vi "SpectrometerSpinCoater_v02_StreamMeasurement.vi"() -> ()   [LabVIEW 2020]
uses:
  <instrlib>/Classes/CCD/Abstract_CCD/Abstract_CCD.lvclass
  TypDef/DeviceQueue_Action.ctl
  TypDef/DeviceQueue_TypeDef.ctl
  TypDef/DataQueue_Action.ctl
  TypDef/DataQueue_TypeDef.ctl
  <instrlib>/Classes/CCD/Avantes/Avantes.lvclass
  <vilib>/Utility/error.llb/DialogType.ctl
  <vilib>/Instr/_visa.llb/VISA Configure Serial Port (Instr).vi
  TypDef/TabControl.ctl
panel:
  out "Arduino":bool
  out "NKT":bool
  out "Spectromter":bool
  in  "Abort Button":bool
  in  "Stop Button":bool
  in  "Tab Control":enum32{"Measure", "Settings"}(tab)
  out "Action":string
  in  "Preview":bool
  out "XY Graph":T1(graph)
  in  "Frames for Dark/Ref":dbl=1.0
  in  "StartSpin_Button":bool
  out "Overall Time":dbl
  in  "Seconds after Spin Stop":dbl[unit]=0.5
  in  "Program Spin Coater\nSpeed (rpm)          Time (s)":dbl[][](array[numeric])
  in  "Record RefSpec":bool
  in  "Record_Darkspec":bool
  in  "Comments":string="Just for testing"
  in  "File Name":string="Temp"
  in  "Save Path":path=path "C:/Users/Timo/Desktop/SpinCoater/Measurement"
  in  "Seconds to Spin Start":dbl[unit]=1.0
  in  "Calculate Frames":bool=TRUE
  in  "Frames":i32
  out "Frame Rate":dbl[unit]
  in  "Integration Time":dbl[unit]=3e-05
  in  "StartMeasurement_Button":bool
  in  "Speed":dbl
  in  "Milliseconds":dbl
  in  "Debug":bool
  in  "Port Arduino":refnum<visa-resource-name>="COM3"
  out "Error Arduino":bool caption="Error"
  in  "Init_Arduino":bool=TRUE caption="Init"
  out "Caption_Settings_Arduino":string="Arduino"
  out "Caption_Settings_NKT":string="NKT Laser"
  out "Error_Spectromter":bool caption="Error"
  in  "Init_Spectrometer":bool=TRUE caption="Init"
  out "Caption_Settings_Spectrometer":string="Spectromter"
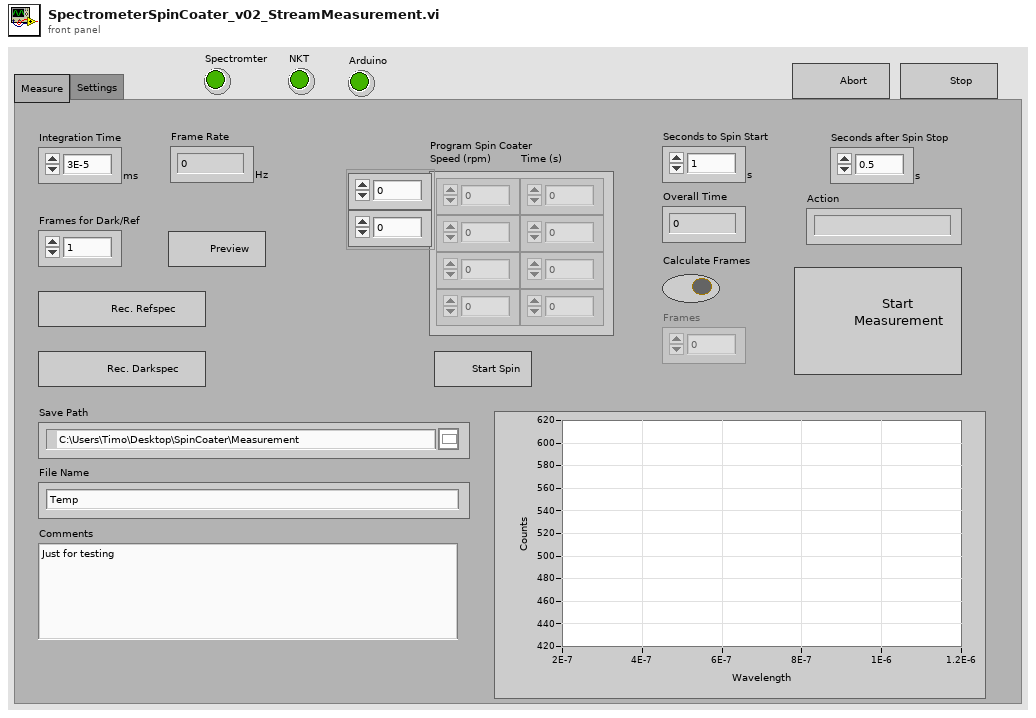
[diagram p1: front panel]
types:
  T1 = cluster{"Wavlength":dbl[unit][], "Image":dbl[]}[]
  T2 = cluster{"Dark":cluster{"Image":dbl[][][], "Frame Size":cluster{"F":i32, "Y":i32, "X":i32}}[], "Ref":cluster{"Image":dbl[][][], "Frame Size":cluster{"F":i32, "Y":i32, "X":i32}}[], "Wavlength":dbl[unit][], "spec":dbl[][]}
  T3 = cluster{"Port Arduino":refnum<visa-resource-name>, "Abstract_CCD.lvclass":refnum<class "Abstract_CCD.lvclass">}
  T4 = typedef "DataQueue_TypeDef.ctl" = cluster{"QueueAction":T5, "Data":cluster{"Image":dbl[][][], "Frame Size":cluster{"F":i32, "Y":i32, "X":i32}}[], "Data_Raw":cluster{"Image":dbl[][][], "Frame Size":cluster{"F":i32, "Y":i32, "X":i32}}[], "Data_Dark":cluster{"Image":dbl[][][], "Frame Size":cluster{"F":i32, "Y":i32, "X":i32}}[], "Data_Ref":cluster{"Image":dbl[][][], "Frame Size":cluster{"F":i32, "Y":i32, "X":i32}}[], "Device Information":string[], "Numeric Control":dbl, "Boolean":bool, "Wavelength":dbl[unit][], "Time":dbl[], "Time Stamp":timestamp, "Numeric Control 2":dbl, "TabControl":T6}
  T5 = typedef "DataQueue_Action.ctl" = enum16{"TimeOut", "Close_Program", "Abort", "Stop_Measurement", "Measure_InSituSpinCoating", "Measure_Spectrum", "Measure_SpectrumAdvanced", "Measure_SpectralStability", "Save_InSitu", "Save_SpectralStability", "Set_Ref", "Set_Dark", "Set_Wavelength", "Spectrometer_Measure", "Spectrometer_Preview", "Transfer_Settings"}
  T6 = typedef "TabControl.ctl" = enum16{"Measure", "Spectral Stability", "Settings"}
  T7 = typedef "DeviceQueue_TypeDef.ctl" = cluster{"QueueAction":T8, "Numeric 1":dbl, "Numeric 2":dbl, "Boolean 1":bool, "Boolean 2":bool, "Spin Program":dbl[][], "Spin Prg v07":cluster{"Speed (rpm)":dbl, "Time (s)":dbl, "Acc (rpm/s)":dbl}[], "Time Stamp":timestamp, "TabControl":T6}
  T8 = typedef "DeviceQueue_Action.ctl" = enum16{"TimeOut", "Wait", "Close_Program", "Abort", "Spectrometer_Init", "Spectrometer_Close", "Spectrometer_DeviceInformation", "Spectrometer_Measure", "Spectrometer_MeasureAdvanced", "Spectrometer_Preview", "Spectrometer_Abort", "Spectrometer_StartMeasurement", "Spectrometer_GetData", "Spectrometer_StopMeasurement", "Spectrometer_SetIntegrationTime", "Spectrometer_SetFrames", "Spectrometer_SetDarkspec", "Spectrometer_SetReference", "Spectrometer_SetTriggerMode", "Laser_Init", "Laser_Close", "Arduino_Init", "Arduino_Close", "Arduino_LoadProgram", "Arduino_StartProgram", "Arduino_SetSpeed", "Arduino_SetMillis", "Arduino_StopSpin", "Arduino_Shutter_SetPosition", "Arduino_Shutter_Close", "Arduino_Shutter_Open", "Measure_InSitu", "Measure_Spectrum", "Measure_InSituAdvanced", "Measure_SpectralStability", "Measure_Stop"}
  T9 = typedef "DataQueue_Action.ctl" = enum16{"TimeOut", "Close_Program", "Stop_Measurement", "Measure_InSituSpinCoating", "Save_Data", "Set_Ref", "Set_Dark", "Set_Wavelength", "Spectrometer_Measure", "Transfer_Settings"}
  T10 = enum16{"open", "replace", "create", "open or create", "replace or create", "replace or create with confirmation"}
  T11 = cluster{"Image":dbl[][][], "Frame Size":cluster{"F":i32, "Y":i32, "X":i32}}[]
  T12 = cluster{"Image":dbl[][][], "Frame Size":cluster{"F":i32, "Y":i32, "X":i32}}
  T13 = cluster{"Image":dbl[], "Image":dbl[], dbl[], "Numeric Control":dbl, "Numeric Control 2":dbl}
  T14 = typedef "DialogType.ctl" = u16
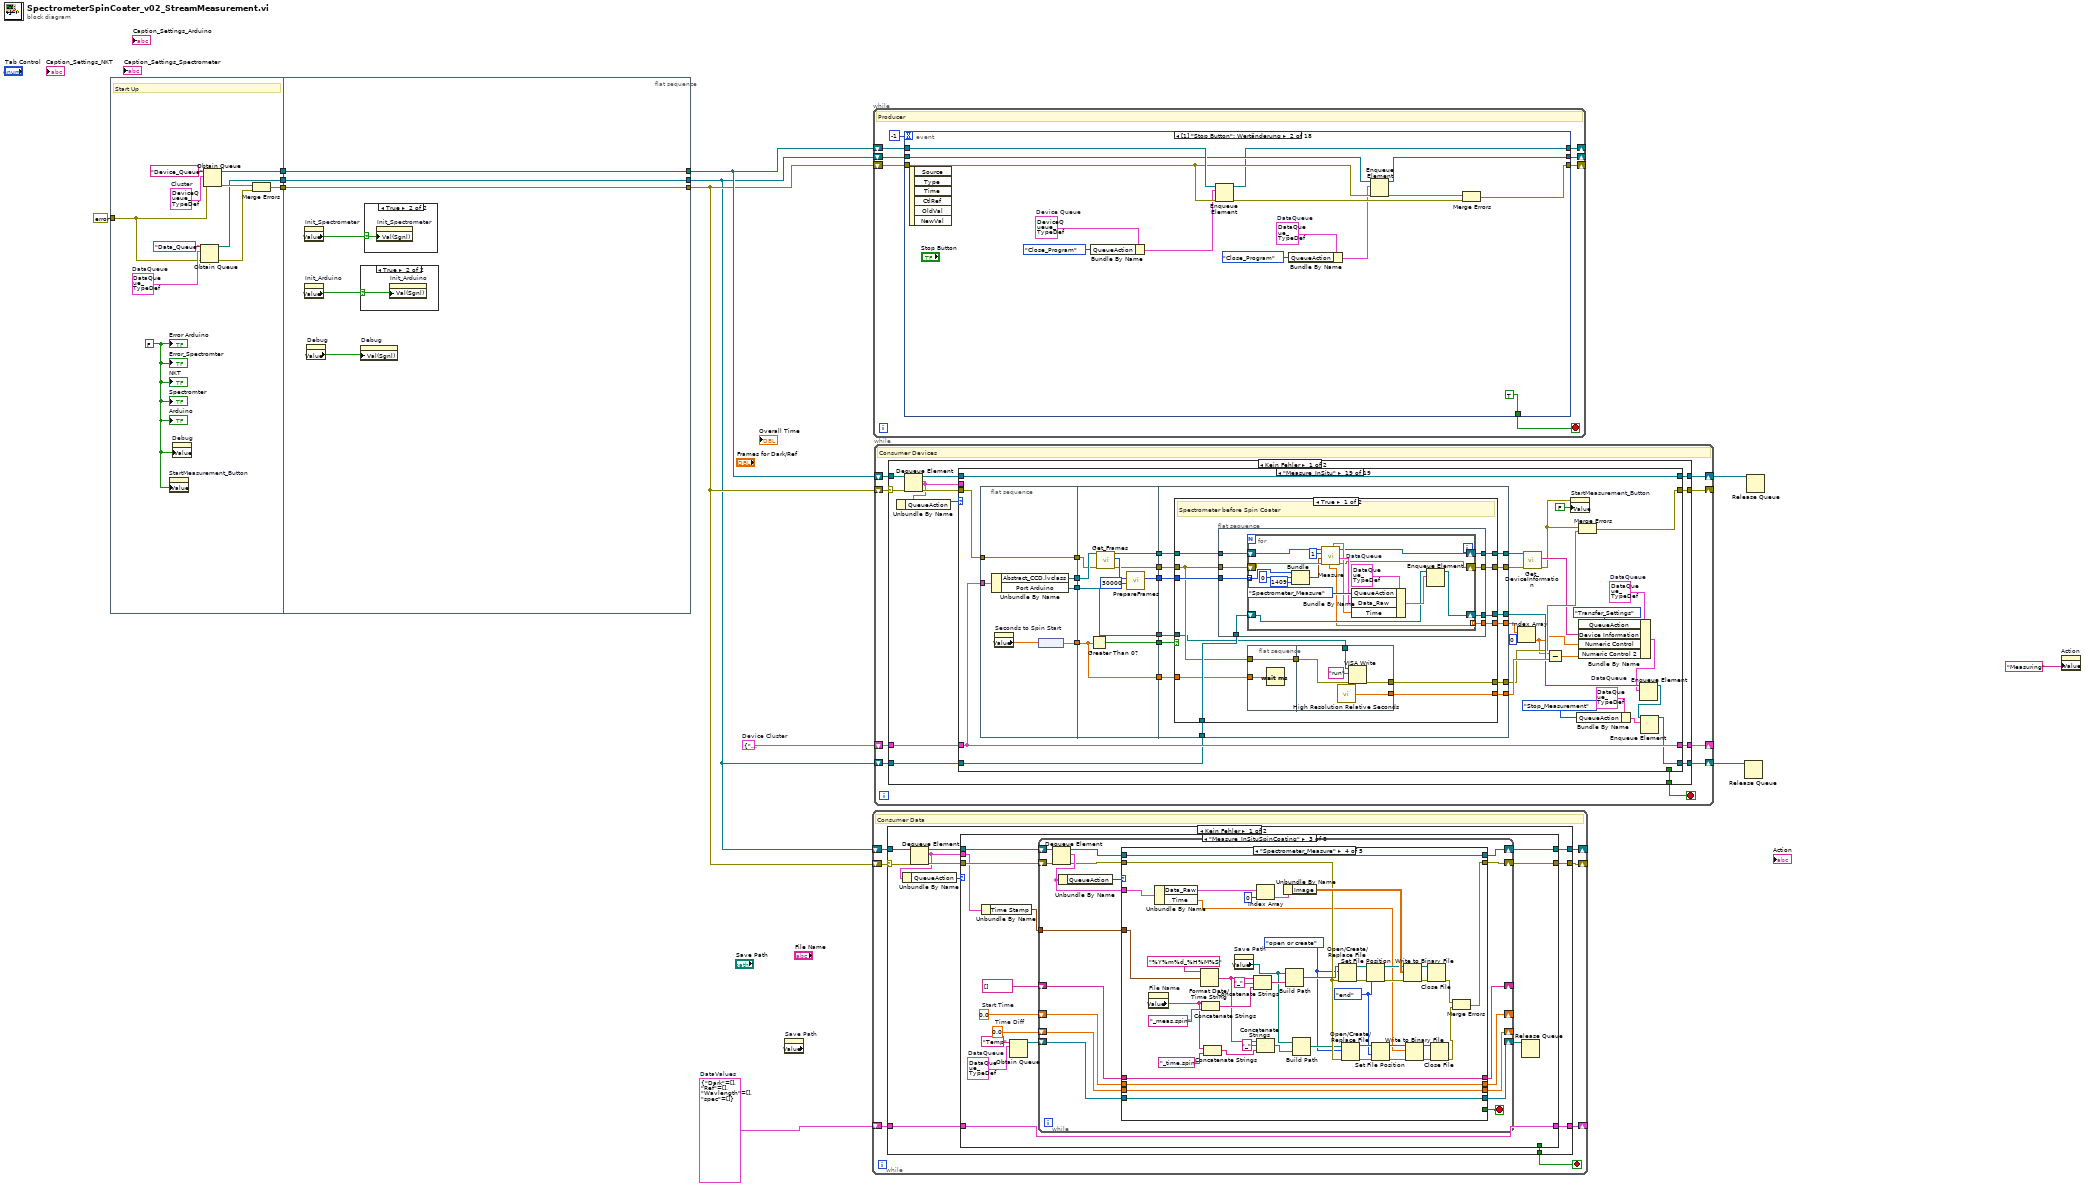
[diagram p0: block diagram]
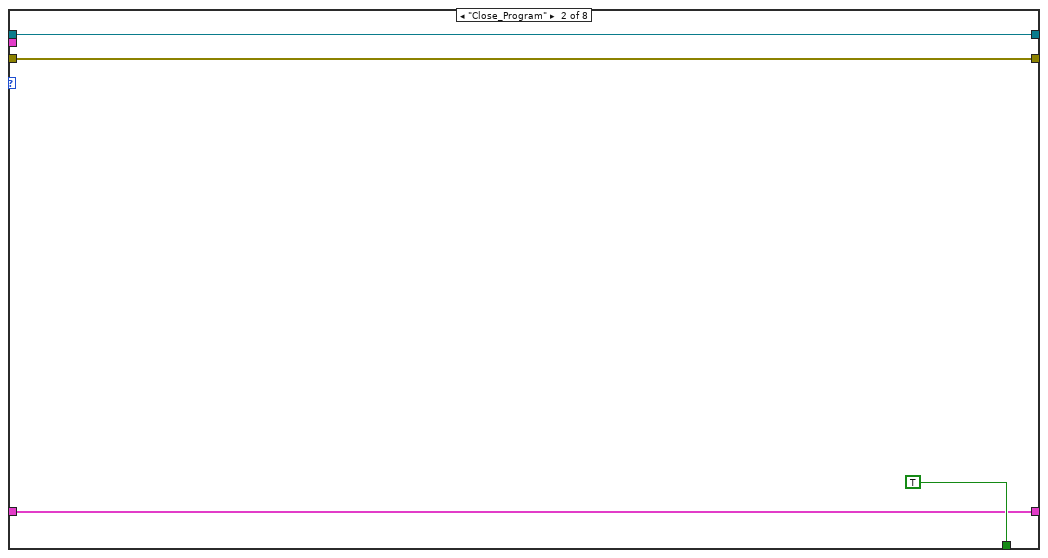
[diagram p5: hidden frame]
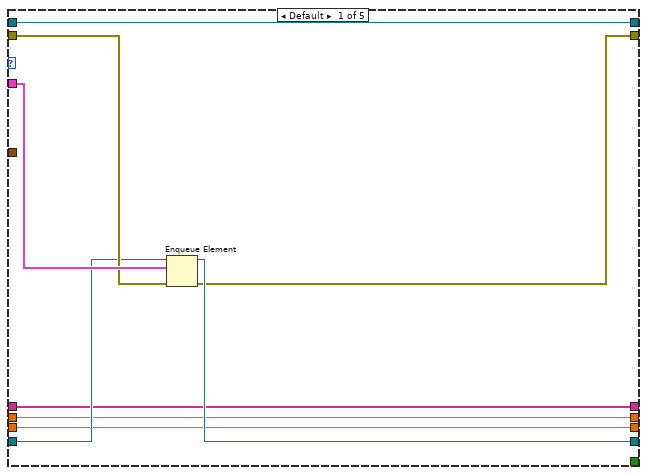
[diagram p6: hidden frame]
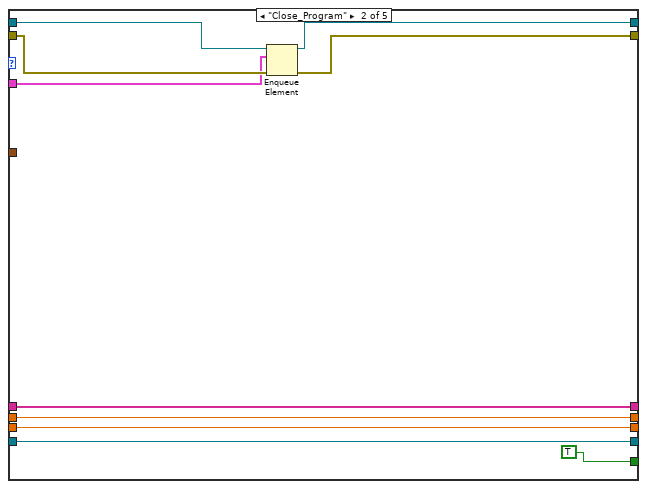
[diagram p7: hidden frame]
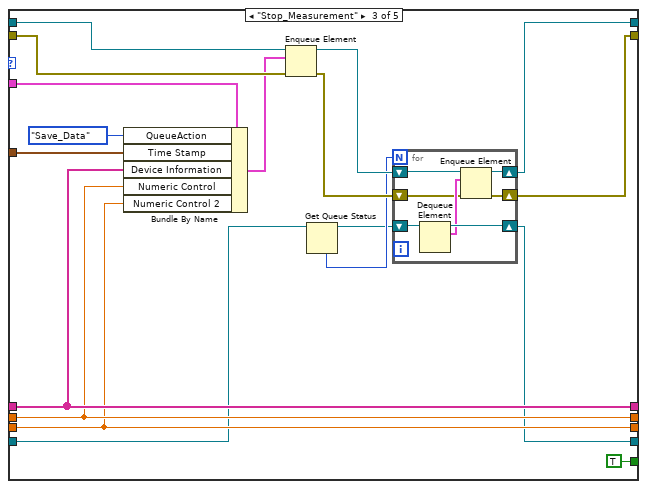
[diagram p8: hidden frame]
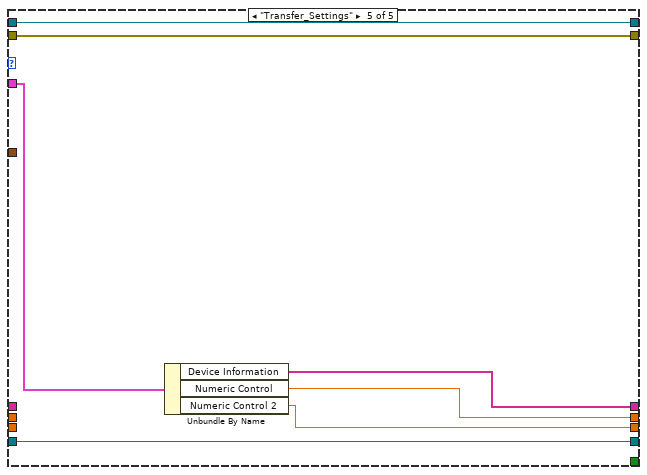
[diagram p9: hidden frame]
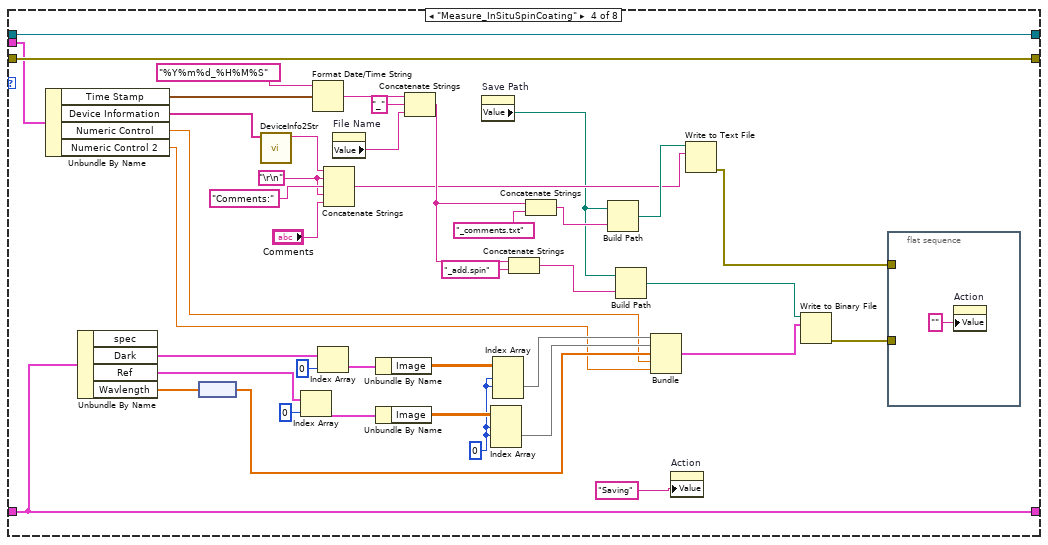
[diagram p10: hidden frame]
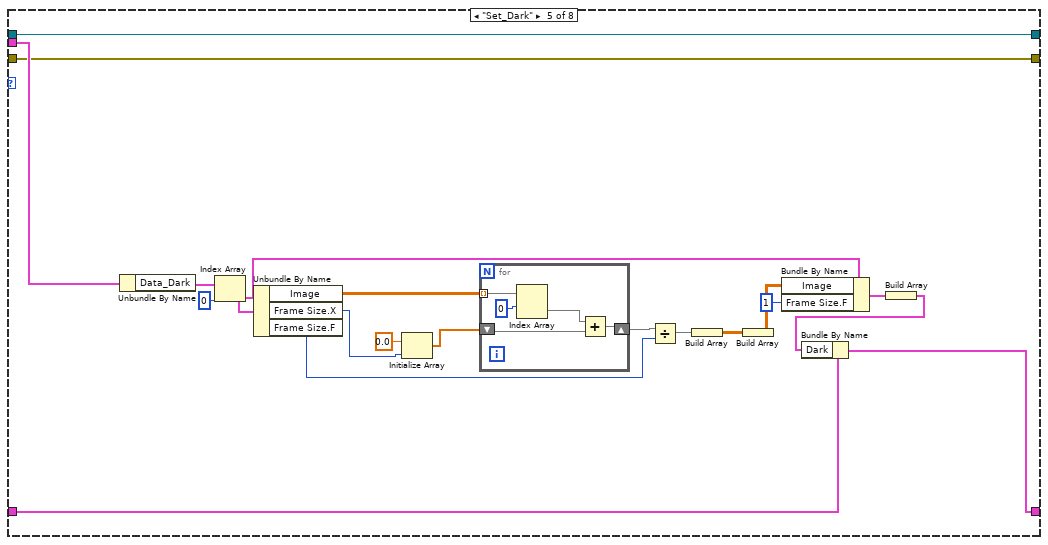
[diagram p11: hidden frame]
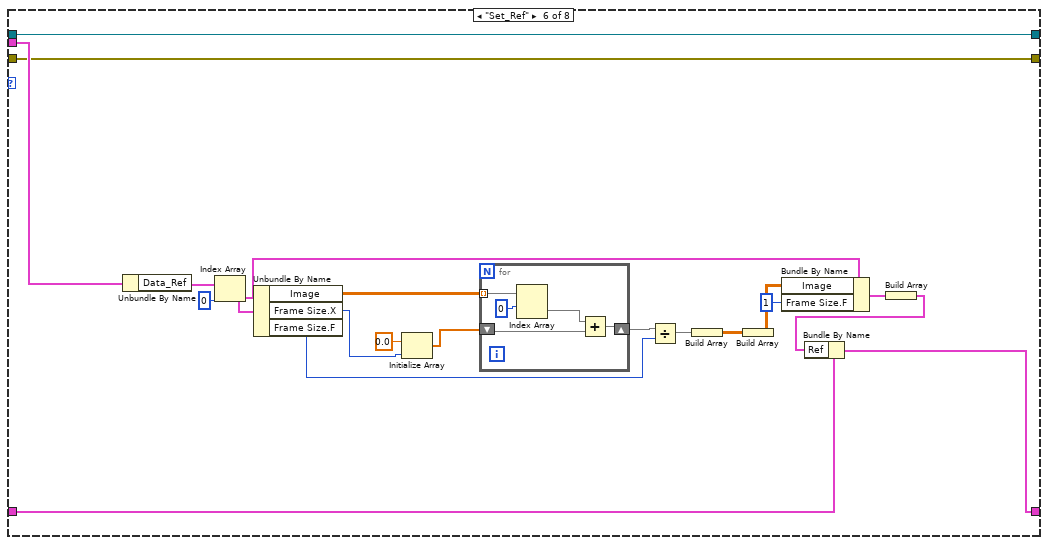
[diagram p12: hidden frame]
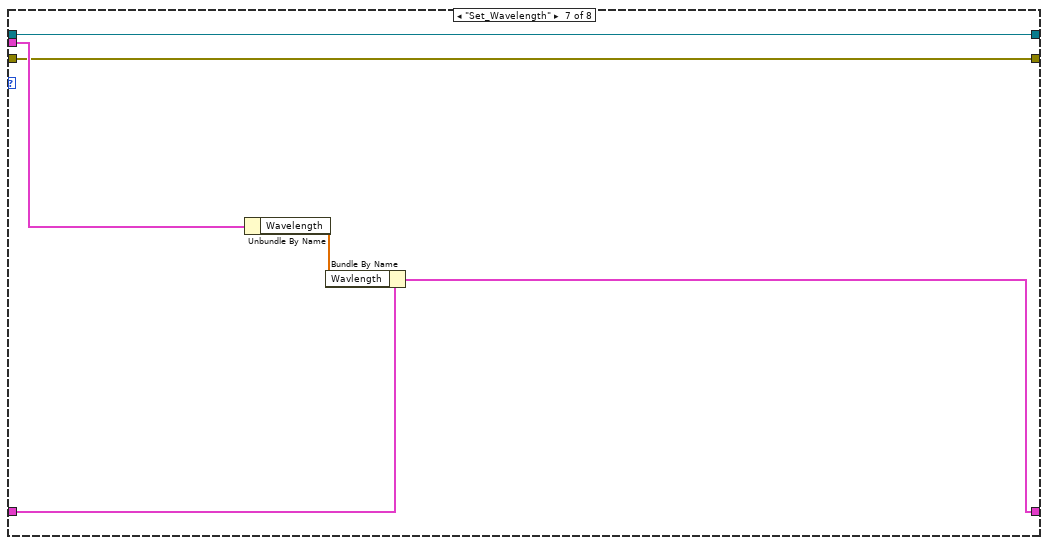
[diagram p13: hidden frame]
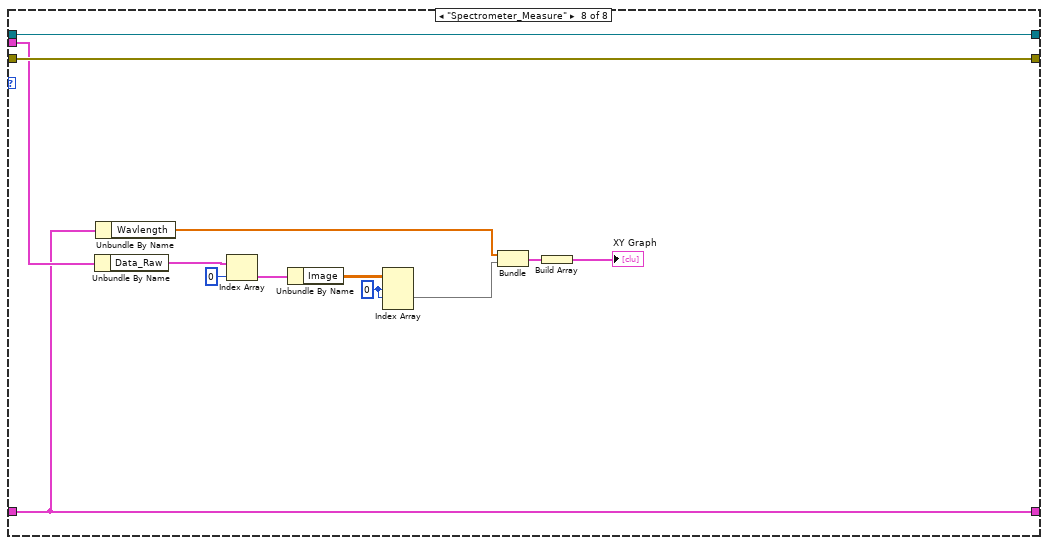
[diagram p14: hidden frame]
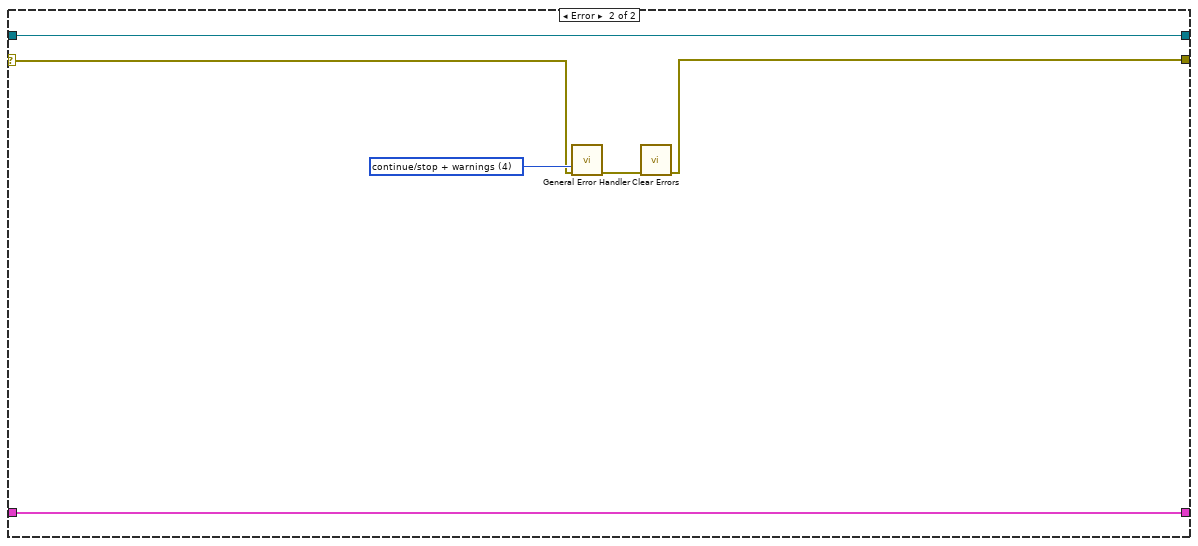
[diagram p15: hidden frame]
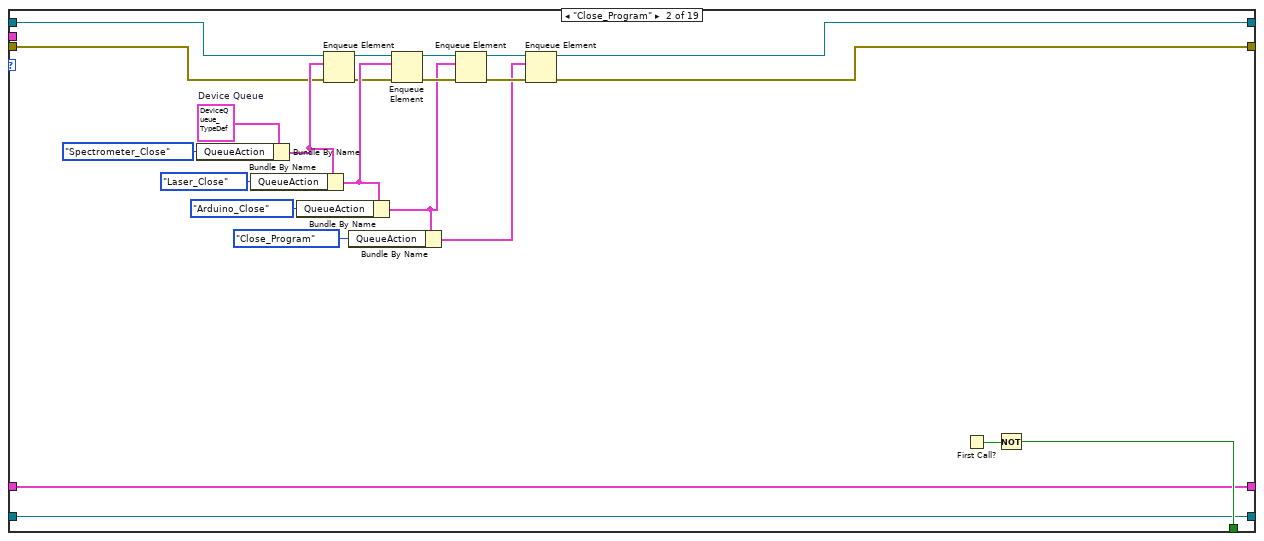
[diagram p17: hidden frame]
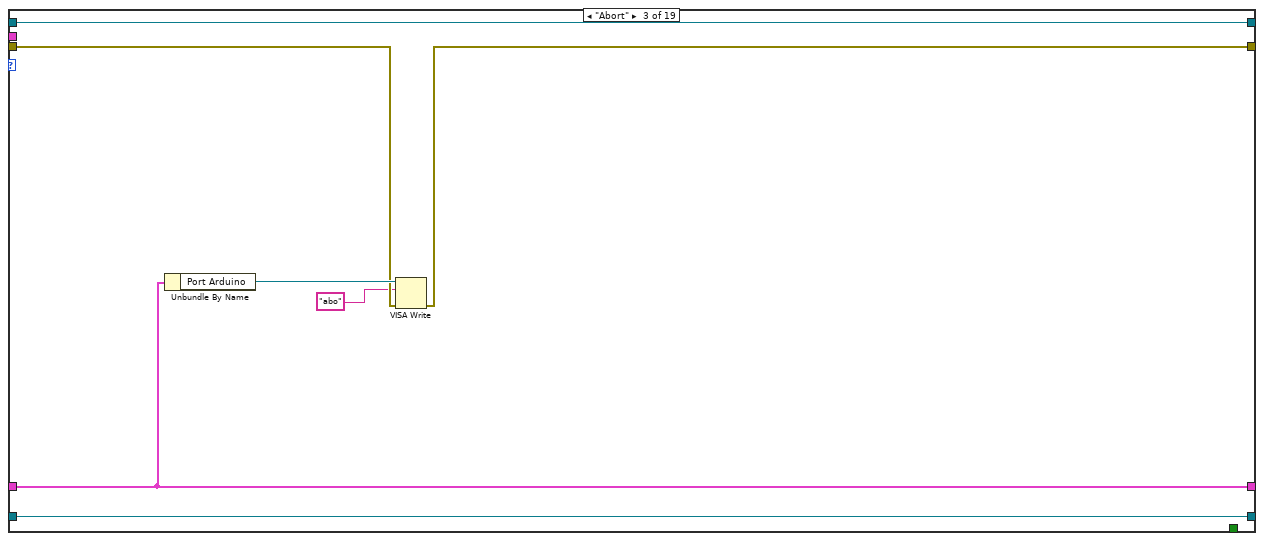
[diagram p18: hidden frame]
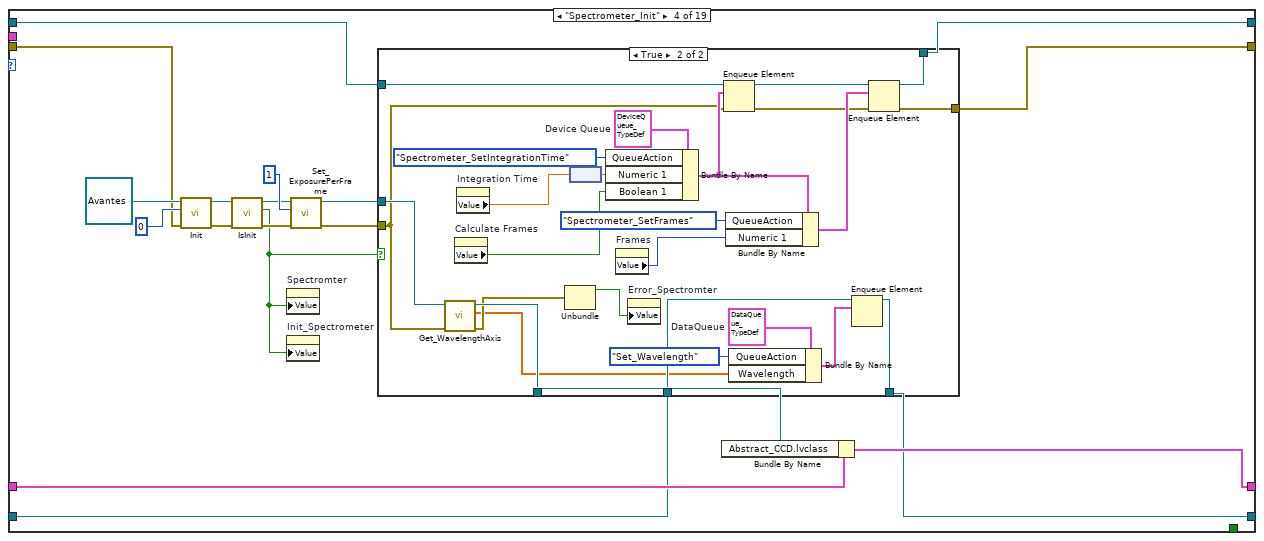
[diagram p19: hidden frame]
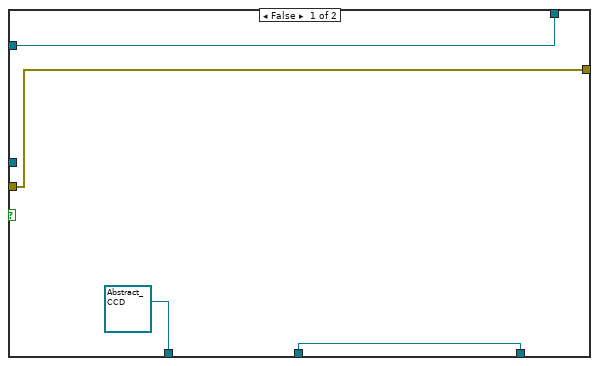
[diagram p20: hidden frame]
diagram:
  w2 = T2 {"Dark"=[], "Ref"=[], "Wavlength"=[], "spec"=[]}  # DataValues
  w7 = T3 {"Port Arduino"="", "Abstract_CCD.lvclass"=refnum}  # Device Cluster
  n1 = flat-sequence {
    tunnel: errorcluster {"status"=FALSE, "code"=0, "source"=""} ("error constant") -> [w18]
    tunnel: [w21] -> w11
    tunnel: [w15] -> w10
    tunnel: [w14] -> w9
    tunnel: w11 -> [w27]
    tunnel: w10 -> [w26]
    tunnel: w9 -> [w25]
    tunnel: [w27] -> w8
    tunnel: [w26] -> w3
    tunnel: [w25] -> w4
    frame #0 {
      w19 = T4 {"QueueAction"=enum."TimeOut", "Data"=[], "Data_Raw"=[], "Data_Dark"=[], "Data_Ref"=[], "Device Information"=[], "Numeric Control"=0.0, "Boolean"=FALSE, "Wavelength"=[], "Time"=[], "Time Stamp"=timestamp(0 s since 1904-01-01), "Numeric Control 2"=0.0, "TabControl"=enum."Measure"}  # DataQueue
      w22 = T7 {"QueueAction"=enum."TimeOut", "Numeric 1"=0.0, "Numeric 2"=0.0, "Boolean 1"=FALSE, "Boolean 2"=FALSE, "Spin Program"=[], "Spin Prg v07"=[], "Time Stamp"=timestamp(0 s since 1904-01-01), "TabControl"=enum."Measure"}  # Cluster
      w13 = FALSE ("Error Arduino")
      # "Start Up"
      n2 = property on="StartMeasurement_Button" class="Bool. (strikt)"("Value"=w13) -> ()  [unwired: 2 in, 2 out]
      n3 = property on="Debug" class="Bool. (strikt)"("Value"=w13) -> ()  [unwired: 2 in, 2 out]
      n4 = Obtain Queue(name (unnamed)="Data_Queue", element data type=w19, error in (no error)=w18) -> (queue out=w15:refnum<queue>, error out=w16:errorcluster)  [unwired: 2 in, 1 out]
      n5 = Obtain Queue(name (unnamed)="Device_Queue", element data type=w22, error in (no error)=w18) -> (queue out=w21:refnum<queue>, error out=w17:errorcluster)  [unwired: 2 in, 1 out]
      n6 = Merge Errors(w17, w16) -> (w14:errorcluster)
      "Error_Spectromter" <- w13
      "Error Arduino" <- w13
      "Spectromter" <- w13
      "NKT" <- w13
      "Arduino" <- w13
    }
    frame #1 {
      n7 = property on="Init_Spectrometer" class="Bool. (strikt)"() -> ("Value"=w29:bool)  [unwired: 2 in, 2 out]
      n8 = property on="Init_Arduino" class="Bool. (strikt)"() -> ("Value"=w28:bool)  [unwired: 2 in, 2 out]
      n9 = property on="Debug" class="Bool. (strikt)"() -> ("Value"=w24:bool)  [unwired: 2 in, 2 out]
      n10 = case shown="True" w28 {
        selector: w28 -> [_ w30]
        frame False {
        }
        frame True {
          n11 = property on="Init_Arduino" class="Bool. (strikt)"("Val(Sgnl)"=w30) -> ()  [unwired: 2 in, 2 out]
        }
      }
      n12 = property on="Debug" class="Bool. (strikt)"("Val(Sgnl)"=w24) -> ()  [unwired: 2 in, 2 out]
      n13 = case shown="True" w29 {
        selector: w29 -> [_ w31]
        frame False {
        }
        frame True {
          n14 = property on="Init_Spectrometer" class="Bool. (strikt)"("Val(Sgnl)"=w31) -> ()  [unwired: 2 in, 2 out]
        }
      }
    }
  }
  n15 = property on="Save Path" class="Pfad" props=["Value"]() -> ()  [unwired: 2 in, 3 out]
  n16 = while {
    shift-right: [w32] -> _
    shift-left: w4 -> [w38]
    shift-right: [w33] -> _
    shift-left: w3 -> [w37]
    shift-right: [w34] -> _
    shift-left: w2 -> [w36]
    stop <- w35 stop-if-true
    # "Consumer Data"
    n17 = case shown="Kein Fehler" w38 {
      selector: w38 -> [w49 w298]
      tunnel: w37 -> [w48 w299]
      tunnel: w36 -> [w46 w296]
      tunnel: [w45 _] -> w35
      tunnel: [w44 w296] -> w34
      tunnel: [w43 w299] -> w33
      tunnel: [w41 w297] -> w32
      frame No Error {
        n18 = Dequeue Element(queue=w48, error in (no error)=w49) -> (queue out=w42:refnum<queue>, element=w39:T4, error out=w40:errorcluster)  [unwired: 1 in, 1 out]
        n19 = Unbundle By Name(w39) -> ("QueueAction"=w47:T5)
        n20 = case shown="\"Measure_InSituSpinCoating\"" w47 {
          tunnel: w46 -> [w50 w55 w60 w194 w246 w271 w281 w292]
          tunnel: [_ TRUE _ _ _ _ _ _] -> w45
          tunnel: [w50 w55 w60 w194 w242 w267 w280 w292] -> w44
          tunnel: [w52 w54 w70 w225 w243 w268 w277 w295] -> w43
          tunnel: w42 -> [w52 w54 w68 w225 w243 w268 w277 w295]
          tunnel: [w51 w53 w69 w224 w244 w269 w278 w294] -> w41
          tunnel: w40 -> [w51 w53 w67 w224 w244 w269 w278 w294]
          tunnel: w39 -> [_ _ w62 w210 w245 w270 w279 w293]
          frame "TimeOut", Default {
          }
          frame "Close_Program" {
          }
          frame "Measure_InSituSpinCoating" {
            w58 = 0.0  # Time Diff
            w59 = 0.0  # Start Time
            w65 = T4 {"QueueAction"=enum."TimeOut", "Data"=[], "Data_Raw"=[], "Data_Dark"=[], "Data_Ref"=[], "Device Information"=[], "Numeric Control"=0.0, "Boolean"=FALSE, "Wavelength"=[], "Time"=[], "Time Stamp"=timestamp(0 s since 1904-01-01), "Numeric Control 2"=0.0, "TabControl"=enum."Measure"}  # DataQueue
            n21 = Unbundle By Name(w62) -> ("Time Stamp"=w61:timestamp)
            n22 = Obtain Queue(name (unnamed)="Temp", element data type=w65) -> (queue out=w64:refnum<queue>)  [unwired: 3 in, 2 out]
            n23 = while {
              shift-right: [w79] -> w70
              shift-left: w68 -> [w88]
              shift-right: [w80] -> w69
              shift-left: w67 -> [w87]
              shift-right: [w81] -> w63
              shift-left: w64 -> [w82]
              tunnel: w61 -> [w71]
              shift-right: [w74] -> _
              shift-left: w59 -> [w76]
              shift-right: [w75] -> _
              shift-left: w58 -> [w77]
              shift-right: [w72] -> _
              shift-left: string[] [] ("Device Information") -> [w73]
              stop <- w78 stop-if-true
              n24 = Dequeue Element(queue=w88, error in (no error)=w87) -> (queue out=w83:refnum<queue>, element=w85:T4, error out=w84:errorcluster)  [unwired: 1 in, 1 out]
              n25 = Unbundle By Name(w85) -> ("QueueAction"=w86:T5)
              n26 = case shown="\"Spectrometer_Measure\"" w86 {
                tunnel: w85 -> [w97 w105 w124 w170 w182]
                tunnel: w84 -> [w96 w106 w119 w149 w177]
                tunnel: w83 -> [w92 w107 w118 w167 w178]
                tunnel: w82 -> [w95 w102 w113 w138 w183]
                tunnel: [w94 w102 w110 w138 w183] -> w81
                tunnel: [w93 w103 w109 w139 w177] -> w80
                tunnel: [w92 w104 w108 w167 w178] -> w79
                tunnel: [_ TRUE TRUE _ _] -> w78
                tunnel: w77 -> [w89 w99 w120 w134 _]
                tunnel: w76 -> [w90 w100 w121 w135 _]
                tunnel: [w89 w99 w120 w134 w179] -> w75
                tunnel: [w90 w100 w121 w135 w180] -> w74
                tunnel: w73 -> [w91 w98 w122 w136 _]
                tunnel: [w91 w98 w122 w136 w181] -> w72
                tunnel: w71 -> [_ _ w123 w172 _]
                frame Default {
                  n27 = Enqueue Element(queue=w95, element=w97, error in (no error)=w96) -> (queue out=w94:refnum<queue>, error out=w93:errorcluster)  [unwired: 1 in, 1 out]
                }
                frame "Close_Program" {
                  n28 = Enqueue Element(queue=w107, element=w105, error in (no error)=w106) -> (queue out=w104:refnum<queue>, error out=w103:errorcluster)  [unwired: 1 in, 1 out]
                }
                frame "Stop_Measurement" {
                  n29 = Bundle By Name(cluster=w124, "QueueAction"=DataQueue_Action."Save_Data", "Time Stamp"=w123, "Device Information"=w122, "Numeric Control"=w121, "Numeric Control 2"=w120) -> (w117:T4)
                  n30 = Enqueue Element(queue=w118, element=w117, error in (no error)=w119) -> (queue out=w115:refnum<queue>, error out=w114:errorcluster)  [unwired: 1 in, 1 out]
                  n31 = Get Queue Status(queue=w113) -> (queue out=w111:refnum<queue>, # elements in queue=w112:i32)  [unwired: 2 in, 6 out]
                  n32 = for {
                    N: w112 -> [_]
                    shift-right: [w131] -> w110
                    shift-left: w111 -> [w132]
                    shift-right: [w128] -> w108
                    shift-left: w115 -> [w129]
                    shift-right: [w126] -> w109
                    shift-left: w114 -> [w127]
                    n33 = Dequeue Element(queue=w132) -> (queue out=w131:refnum<queue>, element=w130:T4)  [unwired: 2 in, 2 out]
                    n34 = Enqueue Element(queue=w129, element=w130, error in (no error)=w127) -> (queue out=w128:refnum<queue>, error out=w126:errorcluster)  [unwired: 1 in, 1 out]
                  }
                }
                frame "Spectrometer_Measure" {
                  w133 = T10."open or create" ("operation (0:open)")
                  w137 = enum16{"start", "end", "current"}."end" ("from (0:start)")
                  n35 = property on="File Name" class="Str"() -> ("Value"=w169:string)  [unwired: 2 in, 2 out]
                  n36 = Unbundle By Name(w170) -> ("Data_Raw"=w160:T11, "Time"=w148:dbl[])
                  n37 = Format Date/Time String(time format string (%c)="%Y%m%d_%H%M%S", seconds (now)=w172) -> (date/time string=w147:string)  [unwired: 1 in]
                  n38 = Concatenate Strings(w169, "_meas.spin" ("string")) -> (w173:string)
                  n39 = Concatenate Strings(w169, "_time.spin" ("string")) -> (w145:string)
                  n40 = property on="Save Path" class="Pfad"() -> ("Value"=w143:path)  [unwired: 2 in, 2 out]
                  n41 = Concatenate Strings(w147, "_" ("string"), w173) -> (w171:string)
                  n42 = Index Array(array=w160, index=0) -> (element=w159:T12)
                  n43 = Concatenate Strings(w147, "_" ("string"), w145) -> (w144:string)
                  n44 = Unbundle By Name(w159) -> ("Image"=w157:dbl[][][])
                  n45 = Build Path(base path=w143, name or relative path=w171) -> (appended path=w150:path)
                  n46 = Build Path(base path=w143, name or relative path=w144) -> (appended path=w142:path)
                  n47 = Open/Create/Replace File(file path (use dialog)=w150, error in=w149, operation (0:open)=w133) -> (refnum out=w152:refnum<file>, error out=w151:errorcluster)  [unwired: 3 in, 1 out]
                  n48 = Open/Create/Replace File(file path (use dialog)=w142, error in=w149, operation (0:open)=w133) -> (refnum out=w166:refnum<file>, error out=w161:errorcluster)  [unwired: 3 in, 1 out]
                  n49 = Set File Position(refnum=w152, from (0:start)=w137, error in=w151) -> (refnum out=w156:refnum<file>, error out=w155:errorcluster)  [unwired: 1 in]
                  n50 = Set File Position(refnum=w166, from (0:start)=w137, error in=w161) -> (refnum out=w165:refnum<file>, error out=w162:errorcluster)  [unwired: 1 in]
                  n51 = Write to Binary File(file (use dialog)=w156, data=w157, error in=w155) -> (refnum out=w153:refnum<file>, error out=w154:errorcluster)  [unwired: 3 in, 1 out]
                  n52 = Write to Binary File(file (use dialog)=w165, data=w148, error in=w162) -> (refnum out=w164:refnum<file>, error out=w163:errorcluster)  [unwired: 3 in, 1 out]
                  n53 = Close File(refnum=w153, error in=w154) -> (error out=w141:errorcluster)  [unwired: 1 out]
                  n54 = Close File(refnum=w164, error in=w163) -> (error out=w140:errorcluster)  [unwired: 1 out]
                  n55 = Merge Errors(w141, w140) -> (w139:errorcluster)
                }
                frame "Transfer_Settings" {
                  n56 = Unbundle By Name(w182) -> ("Device Information"=w181:string[], "Numeric Control"=w180:dbl, "Numeric Control 2"=w179:dbl)
                }
              }
            }
            n57 = Release Queue(queue=w63) -> ()  [unwired: 2 in, 3 out]
          }
          frame "Measure_InSituSpinCoating" {
            w196 = "\r\n"
            w214 = 0 ("index (page)")
            n58 = Unbundle By Name(w210) -> ("Time Stamp"=w208:timestamp, "Device Information"=w199:string[], "Numeric Control"=w193:dbl, "Numeric Control 2"=w192:dbl)
            n59 = Unbundle By Name(w194) -> ("Dark"=w221:T11, "Ref"=w219:T11, "Wavlength"=w223:dbl[unit][])  [unwired: 1 out]
            n60 = node(w223) -> (w211:dbl[])
            n61 = call "DeviceInfo2Str.vi"("Device Information"=w199) -> ("String"=w198:string)  [unwired: 10 in]
            n62 = Index Array(array=w219, index=0) -> (element=w217:T12)
            n63 = Format Date/Time String(time format string (%c)="%Y%m%d_%H%M%S", seconds (now)=w208) -> (date/time string=w207:string)  [unwired: 1 in]
            n64 = Index Array(array=w221, index=0) -> (element=w218:T12)
            n65 = Concatenate Strings(w198, w196, "Comments:" ("string"), w196, "Comments") -> (w191:string)
            n66 = property on="File Name" class="Str"() -> ("Value"=w189:string)  [unwired: 2 in, 2 out]
            n67 = Unbundle By Name(w218) -> ("Image"=w216:dbl[][][])
            n68 = Unbundle By Name(w217) -> ("Image"=w215:dbl[][][])
            n69 = Concatenate Strings(w207, "_" ("string"), w189) -> (w205:string)
            n70 = property on="Save Path" class="Pfad"() -> ("Value"=w188:path)  [unwired: 2 in, 2 out]
            n71 = Index Array(array=w215, index (dim 0)=w214, index (dim 1)=w214) -> (element=w212:dbl[])  [unwired: 1 in]
            n72 = Index Array(array=w216, index (dim 0)=w214, index (dim 1)=w214) -> (element=w213:dbl[])  [unwired: 1 in]
            n73 = Concatenate Strings(w205, "_add.spin" ("string")) -> (w203:string)
            n74 = Concatenate Strings(w205, "_comments.txt" ("string")) -> (w202:string)
            n75 = Build Path(base path=w188, name or relative path=w202) -> (appended path=w201:path)
            n76 = Build Path(base path=w188, name or relative path=w203) -> (appended path=w187:path)
            n77 = Bundle("Image"=w213, "Image"=w212, w211, "Numeric Control"=w193, "Numeric Control 2"=w192) -> (w186:T13)  [unwired: 1 in]
            n78 = property on="Action" class="Str"("Value"="Saving" ("Action")) -> ()  [unwired: 2 in, 2 out]
            n79 = Write to Text File(file (use dialog)=w201, text=w191) -> (error out=w185:errorcluster)  [unwired: 2 in, 2 out]
            n80 = Write to Binary File(file (use dialog)=w187, data=w186) -> (error out=w184:errorcluster)  [unwired: 4 in, 2 out]
            n81 = flat-sequence {
              tunnel: w185 -> [_]
              tunnel: w184 -> [_]
              frame #0 {
                n82 = property on="Action" class="Str"("Value"="" ("Action")) -> ()  [unwired: 2 in, 2 out]
              }
            }
          }
          frame "Set_Dark" {
            n83 = Unbundle By Name(w245) -> ("Data_Dark"=w232:T11)
            n84 = Index Array(array=w232, index=0) -> (element=w231:T12)
            n85 = Unbundle By Name(w231) -> ("Image"=w240:dbl[][][], "Frame Size.X"=w238:i32, "Frame Size.F"=w235:i32)
            n86 = Initialize Array(0.0 ("element"), w238) -> (w237:dbl[])
            n87 = for {
              tunnel: w240 -> [w251] mode=indexing
              shift-right: [w247] -> w236
              shift-left: w237 -> [w248]
              n88 = Index Array(array=w251, index (row)=0) -> (element=w249:dbl[])  [unwired: 1 in]
              n89 = Add(x=w249, y=w248) -> (x+y=w247:dbl[])
            }
            n90 = Divide(x=w236, y=w235) -> (x/y=w234:dbl[])
            n91 = Build Array(w234) -> (w233:dbl[][])
            n92 = Build Array(w233) -> (w230:dbl[][][])
            n93 = Bundle By Name(cluster=w231, "Image"=w230, "Frame Size.F"=1) -> (w228:T12)
            n94 = Build Array(w228) -> (w227:T11)
            n95 = Bundle By Name(cluster=w246, "Dark"=w227) -> (w242:T2)
          }
          frame "Set_Ref" {
            n96 = Unbundle By Name(w270) -> ("Data_Ref"=w257:T11)
            n97 = Index Array(array=w257, index=0) -> (element=w256:T12)
            n98 = Unbundle By Name(w256) -> ("Image"=w265:dbl[][][], "Frame Size.X"=w263:i32, "Frame Size.F"=w260:i32)
            n99 = Initialize Array(0.0 ("element"), w263) -> (w262:dbl[])
            n100 = for {
              tunnel: w265 -> [w276] mode=indexing
              shift-right: [w272] -> w261
              shift-left: w262 -> [w273]
              n101 = Index Array(array=w276, index (row)=0) -> (element=w274:dbl[])  [unwired: 1 in]
              n102 = Add(x=w274, y=w273) -> (x+y=w272:dbl[])
            }
            n103 = Divide(x=w261, y=w260) -> (x/y=w259:dbl[])
            n104 = Build Array(w259) -> (w258:dbl[][])
            n105 = Build Array(w258) -> (w255:dbl[][][])
            n106 = Bundle By Name(cluster=w256, "Image"=w255, "Frame Size.F"=1) -> (w253:T12)
            n107 = Build Array(w253) -> (w252:T11)
            n108 = Bundle By Name(cluster=w271, "Ref"=w252) -> (w267:T2)
          }
          frame "Set_Wavelength" {
            n109 = Unbundle By Name(w279) -> ("Wavelength"=w282:dbl[unit][])
            n110 = Bundle By Name(cluster=w281, "Wavlength"=w282) -> (w280:T2)
          }
          frame "Spectrometer_Measure" {
            w287 = 0 ("index (page)")
            n111 = Unbundle By Name(w293) -> ("Data_Raw"=w291:T11)
            n112 = Unbundle By Name(w292) -> ("Wavlength"=w286:dbl[unit][])
            n113 = Index Array(array=w291, index=0) -> (element=w289:T12)
            n114 = Unbundle By Name(w289) -> ("Image"=w288:dbl[][][])
            n115 = Index Array(array=w288, index (dim 0)=w287, index (dim 1)=w287) -> (element=w285:dbl[])  [unwired: 1 in]
            n116 = Bundle("Wavlength"=w286, "Image"=w285) -> (w284:cluster{"Wavlength":dbl[unit][], "Image":dbl[]})  [unwired: 1 in]
            n117 = Build Array(w284) -> (→"XY Graph":T1)
          }
        }
      }
      frame Error {
        w301 = T14 4 items=["no dialog", "OK message", "continue or stop message", "OK message + warnings", "continue/stop + warnings"] ("type of dialog (OK msg:1)")
        n118 = call <vilib>:"General Error Handler.vi"("type of dialog (OK msg:1)"=w301, "error in (no error)"=w298) -> ("error out"=w300:errorcluster)  [unwired: 9 in, 4 out]
        n119 = call <vilib>:"Clear Errors.vi"("error in (no error)"=w300) -> ("error out"=w297:errorcluster)  [unwired: 5 in, 1 out]
      }
    }
  }
  n120 = while {
    shift-right: [w304] -> _
    shift-left: w8 -> [w302]
    shift-right: [w307] -> _
    shift-left: w3 -> [w308]
    shift-right: [w305] -> _
    shift-left: w4 -> [w306]
    stop <- w303 stop-if-true
    # "Producer"
    n121 = event shown="[1] \"Stop Button\": Wertänderung" {
      selector: _ -> [_ _ _ _ _ _ _ _ _ _ _ _ _ _ _ _ _ _]
      dyn-events: _ -> [_ _ _ _ _ _ _ _ _ _ _ _ _ _ _ _ _ _]
      timeout: -1 -> [_ _ _ _ _ _ _ _ _ _ _ _ _ _ _ _ _ _]
      tunnel: w308 -> [w311 w326 w330 w342 w355 w368 w380 w391 w393 w401 w420 w427 w436 w444 w459 w469 w478 w486]
      tunnel: [w311 w323 w330 w342 w355 w368 w380 w391 w393 w401 w420 w427 w436 w443 w459 w469 w478 w486] -> w307
      tunnel: w306 -> [w310 w325 w332 w340 w352 w367 w378 w386 w392 w398 w418 w426 w434 w450 w456 w468 w477 w485]
      tunnel: [w310 w319 w329 w336 w351 w365 w376 w385 w392 w396 w417 w424 w433 w442 w457 w465 w474 w485] -> w305
      tunnel: w302 -> [w312 w327 w333 w341 w354 w369 w379 w388 w394 w399 w421 w428 w437 w452 w460 w470 w479 w487]
      tunnel: [w312 w324 w331 w337 w353 w366 w377 w387 w394 w400 w419 w425 w435 w451 w458 w466 w475 w487] -> w304
      tunnel: [_ TRUE _ _ _ _ _ _ _ _ _ _ _ _ _ _ _ _] -> w303
      event Timeout {
        n122 = event-data() -> ()  [unwired: 1 in, 3 out]
      }
      event "Stop Button": Value Change {
        w315 = T4 {"QueueAction"=enum."TimeOut", "Data"=[], "Data_Raw"=[], "Data_Dark"=[], "Data_Ref"=[], "Device Information"=[], "Numeric Control"=0.0, "Boolean"=FALSE, "Wavelength"=[], "Time"=[], "Time Stamp"=timestamp(0 s since 1904-01-01), "Numeric Control 2"=0.0, "TabControl"=enum."Measure"}  # DataQueue
        w318 = T7 {"QueueAction"=enum."TimeOut", "Numeric 1"=0.0, "Numeric 2"=0.0, "Boolean 1"=FALSE, "Boolean 2"=FALSE, "Spin Program"=[], "Spin Prg v07"=[], "Time Stamp"=timestamp(0 s since 1904-01-01), "TabControl"=enum."Measure"}  # Device Queue
        n123 = event-data() -> ()  [unwired: 1 in, 6 out]
        n124 = Bundle By Name(cluster=w318, "QueueAction"=DeviceQueue_Action."Close_Program") -> (w316:T7)
        n125 = Enqueue Element(queue=w327, element=w316, error in (no error)=w325) -> (queue out=w324:refnum<queue>, error out=w320:errorcluster)  [unwired: 1 in, 1 out]
        n126 = Bundle By Name(cluster=w315, "QueueAction"=DataQueue_Action."Close_Program") -> (w313:T4)
        n127 = Enqueue Element(queue=w326, element=w313, error in (no error)=w325) -> (queue out=w323:refnum<queue>, error out=w321:errorcluster)  [unwired: 1 in, 1 out]
        n128 = Merge Errors(w321, w320) -> (w319:errorcluster)
      }
      event "Abort Button": Value Change {
        w335 = T7 {"QueueAction"=enum."TimeOut", "Numeric 1"=0.0, "Numeric 2"=0.0, "Boolean 1"=FALSE, "Boolean 2"=FALSE, "Spin Program"=[], "Spin Prg v07"=[], "Time Stamp"=timestamp(0 s since 1904-01-01), "TabControl"=enum."Measure"}  # Device Queue
        # "At the moment just spin coater in non in-situ measurements can be stopped"
        n129 = event-data() -> ()  [unwired: 1 in, 6 out]
        n130 = Bundle By Name(cluster=w335, "QueueAction"=DeviceQueue_Action."Abort") -> (w334:T7)
        n131 = Enqueue Element(queue=w333, element=w334, error in (no error)=w332) -> (queue out=w331:refnum<queue>, error out=w329:errorcluster)  [unwired: 1 in, 1 out]
      }
      event "Init_Spectrometer": Value Change {
        n132 = event-data() -> ()  [unwired: 1 in, 6 out]
        n133 = case shown="False" "Init_Spectrometer" {
          tunnel: [w343 w346] -> w338
          frame True {
            n134 = Bundle By Name(cluster=T7 {"QueueAction"=enum."TimeOut", "Numeric 1"=0.0, "Numeric 2"=0.0, "Boolean 1"=FALSE, "Boolean 2"=FALSE, "Spin Program"=[], "Spin Prg v07"=[], "Time Stamp"=timestamp(0 s since 1904-01-01), "TabControl"=enum."Measure"} ("element"), "QueueAction"=DeviceQueue_Action."Spectrometer_Init") -> (w343:T7)
          }
          frame False {
            n135 = Bundle By Name(cluster=T7 {"QueueAction"=enum."TimeOut", "Numeric 1"=0.0, "Numeric 2"=0.0, "Boolean 1"=FALSE, "Boolean 2"=FALSE, "Spin Program"=[], "Spin Prg v07"=[], "Time Stamp"=timestamp(0 s since 1904-01-01), "TabControl"=enum."Measure"} ("element"), "QueueAction"=DeviceQueue_Action."Spectrometer_Close") -> (w346:T7)
          }
        }
        n136 = Enqueue Element(queue=w341, element=w338, error in (no error)=w340) -> (queue out=w337:refnum<queue>, error out=w336:errorcluster)  [unwired: 1 in, 1 out]
      }
      event "Init_Arduino": Value Change {
        n137 = event-data() -> ("NewVal"=w350:bool)  [unwired: 1 in, 5 out]
        n138 = case shown="True" w350 {
          tunnel: [w356 w359] -> w349
          frame False {
            w358 = T7 {"QueueAction"=enum."TimeOut", "Numeric 1"=0.0, "Numeric 2"=0.0, "Boolean 1"=FALSE, "Boolean 2"=FALSE, "Spin Program"=[], "Spin Prg v07"=[], "Time Stamp"=timestamp(0 s since 1904-01-01), "TabControl"=enum."Measure"}  # Device Queue
            n139 = Bundle By Name(cluster=w358, "QueueAction"=DeviceQueue_Action."Arduino_Close") -> (w356:T7)
          }
          frame True {
            w361 = T7 {"QueueAction"=enum."TimeOut", "Numeric 1"=0.0, "Numeric 2"=0.0, "Boolean 1"=FALSE, "Boolean 2"=FALSE, "Spin Program"=[], "Spin Prg v07"=[], "Time Stamp"=timestamp(0 s since 1904-01-01), "TabControl"=enum."Measure"}  # Device Queue
            n140 = Bundle By Name(cluster=w361, "QueueAction"=DeviceQueue_Action."Arduino_Init") -> (w359:T7)
          }
        }
        n141 = Enqueue Element(queue=w354, element=w349, error in (no error)=w352) -> (queue out=w353:refnum<queue>, error out=w351:errorcluster)  [unwired: 1 in, 1 out]
      }
      event "Program Spin Coater\nSpeed (rpm)          Time (s)": Value Change {
        w371 = T7 {"QueueAction"=enum."TimeOut", "Numeric 1"=0.0, "Numeric 2"=0.0, "Boolean 1"=FALSE, "Boolean 2"=FALSE, "Spin Program"=[], "Spin Prg v07"=[], "Time Stamp"=timestamp(0 s since 1904-01-01), "TabControl"=enum."Measure"}  # Device Queue
        n142 = event-data() -> ("NewVal"=w363:dbl[][])  [unwired: 1 in, 5 out]
        n143 = property on="Integration Time" class="DigWert (strikt)"() -> ("Value"=w362:dbl[unit])  [unwired: 2 in, 2 out]
        n144 = property on="Integration Time" class="DigWert (strikt)"("Val(Sgnl)"=w362) -> ()  [unwired: 2 in, 2 out]
        n145 = Bundle By Name(cluster=w371, "QueueAction"=DeviceQueue_Action."Arduino_LoadProgram", "Spin Program"=w363) -> (w370:T7)
        n146 = Enqueue Element(queue=w369, element=w370, error in (no error)=w367) -> (queue out=w366:refnum<queue>, error out=w365:errorcluster)  [unwired: 1 in, 1 out]
      }
      event "Integration Time": Value Change {
        w382 = T7 {"QueueAction"=enum."TimeOut", "Numeric 1"=0.0, "Numeric 2"=0.0, "Boolean 1"=FALSE, "Boolean 2"=FALSE, "Spin Program"=[], "Spin Prg v07"=[], "Time Stamp"=timestamp(0 s since 1904-01-01), "TabControl"=enum."Measure"}  # Device Queue
        n147 = event-data() -> ("NewVal"=w374:dbl[unit])  [unwired: 1 in, 5 out]
        n148 = node(w374) -> (w373:dbl)
        n149 = property on="Calculate Frames" class="Bool. (strikt)"() -> ("Value"=w372:bool)  [unwired: 2 in, 2 out]
        n150 = Bundle By Name(cluster=w382, "QueueAction"=DeviceQueue_Action."Spectrometer_SetIntegrationTime", "Numeric 1"=w373, "Boolean 1"=w372) -> (w381:T7)
        n151 = Enqueue Element(queue=w379, element=w381, error in (no error)=w378) -> (queue out=w377:refnum<queue>, error out=w376:errorcluster)  [unwired: 1 in, 1 out]
      }
      event "Frames": Value Change {
        w390 = T7 {"QueueAction"=enum."TimeOut", "Numeric 1"=0.0, "Numeric 2"=0.0, "Boolean 1"=FALSE, "Boolean 2"=FALSE, "Spin Program"=[], "Spin Prg v07"=[], "Time Stamp"=timestamp(0 s since 1904-01-01), "TabControl"=enum."Measure"}  # Device Queue
        n152 = event-data() -> ()  [unwired: 1 in, 6 out]
        n153 = Bundle By Name(cluster=w390, "QueueAction"=DeviceQueue_Action."Spectrometer_SetFrames", "Numeric 1"="Frames") -> (w389:T7)
        n154 = Enqueue Element(queue=w388, element=w389, error in (no error)=w386) -> (queue out=w387:refnum<queue>, error out=w385:errorcluster)  [unwired: 1 in, 1 out]
      }
      event "Seconds to Spin Start", "Seconds after Spin Stop": Value Change {
        n155 = event-data() -> ()  [unwired: 1 in, 6 out]
        n156 = property on="Integration Time" class="DigWert (strikt)"() -> ("Value"=w395:dbl[unit])  [unwired: 2 in, 2 out]
        n157 = property on="Integration Time" class="DigWert (strikt)"("Val(Sgnl)"=w395) -> ()  [unwired: 2 in, 2 out]
      }
      event "Calculate Frames": Value Change {
        n158 = event-data() -> ("NewVal"=w402:bool)  [unwired: 1 in, 5 out]
        n159 = case shown="False" w402 {
          tunnel: [0 2] -> w397
          tunnel: w399 -> [w404 w413]
          tunnel: [w404 w411] -> w400
          tunnel: w398 -> [w403 w410]
          tunnel: [w403 w406] -> w396
          frame False {
          }
          frame True {
            w412 = T7 {"QueueAction"=enum."TimeOut", "Numeric 1"=0.0, "Numeric 2"=0.0, "Boolean 1"=FALSE, "Boolean 2"=FALSE, "Spin Program"=[], "Spin Prg v07"=[], "Time Stamp"=timestamp(0 s since 1904-01-01), "TabControl"=enum."Measure"}  # Device Queue
            n160 = property on="Integration Time" class="DigWert (strikt)"() -> ("Value"=w408:dbl[unit])  [unwired: 2 in, 2 out]
            n161 = node(w408) -> (w407:dbl)
            n162 = Bundle By Name(cluster=w412, "QueueAction"=DeviceQueue_Action."Spectrometer_SetIntegrationTime", "Numeric 1"=w407) -> (w414:T7)
            n163 = Enqueue Element(queue=w413, element=w414, error in (no error)=w410) -> (queue out=w411:refnum<queue>, error out=w406:errorcluster)  [unwired: 1 in, 1 out]
          }
        }
        n164 = property on="Frames" class="DigWert (strikt)"("DisabledEnum"=w397) -> ()  [unwired: 2 in, 2 out]
      }
      event "Record RefSpec": Value Change {
        w423 = T7 {"QueueAction"=enum."TimeOut", "Numeric 1"=0.0, "Numeric 2"=0.0, "Boolean 1"=FALSE, "Boolean 2"=FALSE, "Spin Program"=[], "Spin Prg v07"=[], "Time Stamp"=timestamp(0 s since 1904-01-01), "TabControl"=enum."Measure"}  # Device Queue
        n165 = event-data() -> ()  [unwired: 1 in, 6 out]
        n166 = Bundle By Name(cluster=w423, "QueueAction"=DeviceQueue_Action."Spectrometer_SetReference") -> (w422:T7)
        n167 = Enqueue Element(queue=w421, element=w422, error in (no error)=w418) -> (queue out=w419:refnum<queue>, error out=w417:errorcluster)  [unwired: 1 in, 1 out]
      }
      event "Preview": Value Change {
        w431 = T7 {"QueueAction"=enum."TimeOut", "Numeric 1"=0.0, "Numeric 2"=0.0, "Boolean 1"=FALSE, "Boolean 2"=FALSE, "Spin Program"=[], "Spin Prg v07"=[], "Time Stamp"=timestamp(0 s since 1904-01-01), "TabControl"=enum."Measure"}  # Device Queue
        n168 = event-data() -> ()  [unwired: 1 in, 6 out]
        n169 = Bundle By Name(cluster=w431, "QueueAction"=DeviceQueue_Action."Spectrometer_Preview") -> (w430:T7)
        n170 = Enqueue Element(queue=w428, element=w430, error in (no error)=w426) -> (queue out=w425:refnum<queue>, error out=w424:errorcluster)  [unwired: 1 in, 1 out]
      }
      event "Record_Darkspec": Value Change {
        w439 = T7 {"QueueAction"=enum."TimeOut", "Numeric 1"=0.0, "Numeric 2"=0.0, "Boolean 1"=FALSE, "Boolean 2"=FALSE, "Spin Program"=[], "Spin Prg v07"=[], "Time Stamp"=timestamp(0 s since 1904-01-01), "TabControl"=enum."Measure"}  # Device Queue
        n171 = event-data() -> ()  [unwired: 1 in, 6 out]
        n172 = Bundle By Name(cluster=w439, "QueueAction"=DeviceQueue_Action."Spectrometer_SetDarkspec") -> (w438:T7)
        n173 = Enqueue Element(queue=w437, element=w438, error in (no error)=w434) -> (queue out=w435:refnum<queue>, error out=w433:errorcluster)  [unwired: 1 in, 1 out]
      }
      event "StartMeasurement_Button": Value Change {
        w446 = T4 {"QueueAction"=enum."TimeOut", "Data"=[], "Data_Raw"=[], "Data_Dark"=[], "Data_Ref"=[], "Device Information"=[], "Numeric Control"=0.0, "Boolean"=FALSE, "Wavelength"=[], "Time"=[], "Time Stamp"=timestamp(0 s since 1904-01-01), "Numeric Control 2"=0.0, "TabControl"=enum."Measure"}  # DataQueue
        w454 = T7 {"QueueAction"=enum."TimeOut", "Numeric 1"=0.0, "Numeric 2"=0.0, "Boolean 1"=FALSE, "Boolean 2"=FALSE, "Spin Program"=[], "Spin Prg v07"=[], "Time Stamp"=timestamp(0 s since 1904-01-01), "TabControl"=enum."Measure"}  # Device Queue
        n174 = event-data() -> ()  [unwired: 1 in, 6 out]
        n175 = property on="Preview" class="Bool. (strikt)"("Value"=FALSE ("Preview")) -> ()  [unwired: 2 in, 2 out]
        n176 = Bundle By Name(cluster=w454, "QueueAction"=DeviceQueue_Action."Measure_InSitu") -> (w453:T7)
        n177 = Enqueue Element(queue=w452, element=w453, error in (no error)=w450) -> (queue out=w451:refnum<queue>, error out=w441:errorcluster)  [unwired: 1 in, 1 out]
        n178 = Get Date/Time In Seconds() -> (seconds since 1Jan1904=w440:timestamp)
        n179 = Bundle By Name(cluster=w446, "QueueAction"=DataQueue_Action."Measure_InSituSpinCoating", "Time Stamp"=w440) -> (w447:T4)
        n180 = Enqueue Element(queue=w444, element=w447, error in (no error)=w441) -> (queue out=w443:refnum<queue>, error out=w442:errorcluster)  [unwired: 1 in, 1 out]
      }
      event "StartSpin_Button": Value Change {
        w462 = T7 {"QueueAction"=enum."TimeOut", "Numeric 1"=0.0, "Numeric 2"=0.0, "Boolean 1"=FALSE, "Boolean 2"=FALSE, "Spin Program"=[], "Spin Prg v07"=[], "Time Stamp"=timestamp(0 s since 1904-01-01), "TabControl"=enum."Measure"}  # Device Queue
        n181 = event-data() -> ()  [unwired: 1 in, 6 out]
        n182 = Bundle By Name(cluster=w462, "QueueAction"=DeviceQueue_Action."Arduino_StartProgram") -> (w461:T7)
        n183 = Enqueue Element(queue=w460, element=w461, error in (no error)=w456) -> (queue out=w458:refnum<queue>, error out=w457:errorcluster)  [unwired: 1 in, 1 out]
      }
      event "Milliseconds": Value Change {
        w471 = T7 {"QueueAction"=enum."TimeOut", "Numeric 1"=0.0, "Numeric 2"=0.0, "Boolean 1"=FALSE, "Boolean 2"=FALSE, "Spin Program"=[], "Spin Prg v07"=[], "Time Stamp"=timestamp(0 s since 1904-01-01), "TabControl"=enum."Measure"}  # Device Queue
        n184 = event-data() -> ()  [unwired: 1 in, 6 out]
        n185 = Bundle By Name(cluster=w471, "QueueAction"=DeviceQueue_Action."Arduino_SetMillis", "Numeric 1"="Milliseconds") -> (w467:T7)
        n186 = Enqueue Element(queue=w470, element=w467, error in (no error)=w468) -> (queue out=w466:refnum<queue>, error out=w465:errorcluster)  [unwired: 1 in, 1 out]
      }
      event "Speed": Value Change {
        w480 = T7 {"QueueAction"=enum."TimeOut", "Numeric 1"=0.0, "Numeric 2"=0.0, "Boolean 1"=FALSE, "Boolean 2"=FALSE, "Spin Program"=[], "Spin Prg v07"=[], "Time Stamp"=timestamp(0 s since 1904-01-01), "TabControl"=enum."Measure"}  # Device Queue
        n187 = event-data() -> ()  [unwired: 1 in, 6 out]
        n188 = Bundle By Name(cluster=w480, "QueueAction"=DeviceQueue_Action."Arduino_SetSpeed", "Numeric 1"="Speed") -> (w476:T7)
        n189 = Enqueue Element(queue=w479, element=w476, error in (no error)=w477) -> (queue out=w475:refnum<queue>, error out=w474:errorcluster)  [unwired: 1 in, 1 out]
      }
      event "Debug": Value Change {
        n190 = event-data() -> ()  [unwired: 1 in, 6 out]
        n191 = Select(t=u8 0, s="Debug", f=u8 2) -> (s? t:f=w481:u8)
        n192 = property on="Milliseconds" class="DigWert (strikt)"("DisabledEnum"=w481) -> ()  [unwired: 2 in, 2 out]
        n193 = property on="Speed" class="DigWert (strikt)"("DisabledEnum"=w481) -> ()  [unwired: 2 in, 2 out]
      }
    }
  }
  n194 = while {
    shift-right: [w492] -> _
    shift-left: w4 -> [w496]
    shift-right: [w493] -> w6
    shift-left: w8 -> [w495]
    shift-right: [w490] -> w5
    shift-left: w3 -> [w491]
    shift-right: [w488] -> _
    shift-left: w7 -> [w489]
    stop <- w494 stop-if-true
    # "Consumer Devices"
    n195 = case shown="Kein Fehler" w496 {
      selector: w496 -> [w508 w962]
      tunnel: w495 -> [w509 w963]
      tunnel: [w505 _] -> w494
      tunnel: [w504 w963] -> w493
      tunnel: [w502 w959] -> w492
      tunnel: w491 -> [w500 w957]
      tunnel: [w501 w957] -> w490
      tunnel: w489 -> [w499 w958]
      tunnel: [w498 w958] -> w488
      frame No Error {
        n196 = Dequeue Element(queue=w509, error in (no error)=w508) -> (queue out=w507:refnum<queue>, element=w497:T7, error out=w503:errorcluster)  [unwired: 1 in, 1 out]
        n197 = Unbundle By Name(w497) -> ("QueueAction"=w506:T8)
        n198 = case shown="\"Measure_InSitu\"" w506 {
          tunnel: w507 -> [w513 w533 w539 w548 w597 w611 w618 w649 w679 w702 w723 w735 w746 w760 w761 w768 w784 w797 w833]
          tunnel: [_ w535 _ _ _ _ _ _ _ _ _ _ _ _ _ _ _ _ _] -> w505
          tunnel: [w513 w518 w539 w547 w597 w611 w619 w648 w679 w702 w723 w728 w746 w760 w761 w768 w784 w797 w833] -> w504
          tunnel: w503 -> [w512 w517 w540 w559 w598 w610 w633 w655 w677 w693 w714 w743 w750 w759 w763 w775 w785 w796 w828]
          tunnel: [w512 w516 w538 w546 w592 w609 w620 w647 w676 w692 w713 w727 w749 w755 w762 w769 w783 w792 w804] -> w502
          tunnel: [w510 w515 w543 w544 w594 w606 w627 w657 w680 w685 w706 w741 w748 w757 w767 w779 w781 w798 w806] -> w501
          tunnel: w500 -> [w510 w515 w543 w545 w594 w607 w628 w657 w680 w688 w709 w741 w748 w757 w767 w779 w781 w798 w822]
          tunnel: w499 -> [w511 w514 w542 w556 w596 w608 w617 w646 w673 w684 w705 w740 w747 w756 w766 w778 w780 w795 w827]
          tunnel: [w511 w514 w542 w550 w595 w608 w616 w644 w674 w683 w704 w738 w747 w756 w766 w778 w780 w795 w827] -> w498
          tunnel: w497 -> [_ _ _ _ _ _ _ w652 w681 _ _ _ _ w754 _ w776 w782 _ _]
          frame "TimeOut", Default {
          }
          frame "Close_Program" {
            w534 = T7 {"QueueAction"=enum."TimeOut", "Numeric 1"=0.0, "Numeric 2"=0.0, "Boolean 1"=FALSE, "Boolean 2"=FALSE, "Spin Program"=[], "Spin Prg v07"=[], "Time Stamp"=timestamp(0 s since 1904-01-01), "TabControl"=enum."Measure"}  # Device Queue
            n199 = Bundle By Name(cluster=w534, "QueueAction"=DeviceQueue_Action."Spectrometer_Close") -> (w529:T7)
            n200 = Bundle By Name(cluster=w529, "QueueAction"=DeviceQueue_Action."Laser_Close") -> (w527:T7)
            n201 = Bundle By Name(cluster=w527, "QueueAction"=DeviceQueue_Action."Arduino_Close") -> (w521:T7)
            n202 = Enqueue Element(queue=w533, element=w529, error in (no error)=w517) -> (queue out=w531:refnum<queue>, error out=w526:errorcluster)  [unwired: 1 in, 1 out]
            n203 = Bundle By Name(cluster=w521, "QueueAction"=DeviceQueue_Action."Close_Program") -> (w519:T7)
            n204 = Enqueue Element(queue=w531, element=w527, error in (no error)=w526) -> (queue out=w525:refnum<queue>, error out=w524:errorcluster)  [unwired: 1 in, 1 out]
            n205 = Enqueue Element(queue=w525, element=w521, error in (no error)=w524) -> (queue out=w523:refnum<queue>, error out=w522:errorcluster)  [unwired: 1 in, 1 out]
            n206 = Enqueue Element(queue=w523, element=w519, error in (no error)=w522) -> (queue out=w518:refnum<queue>, error out=w516:errorcluster)  [unwired: 1 in, 1 out]
            n207 = First Call?() -> (First Call?: T/F=w536:bool)
            n208 = Not(x=w536) -> (.not. x?=w535:bool)
          }
          frame "Abort" {
            n209 = Unbundle By Name(w542) -> ("Port Arduino"=w541:refnum<visa-resource-name>)
            n210 = VISA Write(VISA resource name=w541, write buffer="abo", error in (no error)=w540) -> (error out=w538:errorcluster)  [unwired: 2 out]
          }
          frame "Spectrometer_Init" {
            n211 = call-dynamic "Init.vi"("error in (no error)"=w559, "Variant"=0, "Avantes in"=refnum<class "Avantes.lvclass"> refnum ("Avantes.lvclass")) -> ("error out"=w558:errorcluster, "Avantes out"=w557:refnum<class "Avantes.lvclass">)  [unwired: 7 in]
            n212 = call-dynamic "IsInit.vi"("error in (no error)"=w558, "Avantes in"=w557) -> ("error out"=w554:errorcluster, "Is Init?"=w553:bool, "Avantes out"=w555:refnum<class "Avantes.lvclass">)  [unwired: 7 in]
            n213 = property on="Spectromter" class="Bool. (strikt)"("Value"=w553) -> ()  [unwired: 2 in, 2 out]
            n214 = property on="Init_Spectrometer" class="Bool. (strikt)"("Value"=w553) -> ()  [unwired: 2 in, 2 out]
            n215 = call-dynamic "Set_ExposurePerFrame.vi"("error in (no error)"=w554, "Exposure per Frame"=1, "Avantes in"=w555) -> ("error out"=w549:errorcluster, "Avantes out"=w552:refnum<class "Avantes.lvclass">)  [unwired: 7 in]
            n216 = case shown="True" w553 {
              tunnel: w552 -> [_ w575]
              tunnel: w549 -> [w564 w573]
              tunnel: [refnum<class "Abstract_CCD.lvclass"> refnum ("Abstract_CCD.lvclass") w574] -> w551
              tunnel: w548 -> [w565 w590]
              tunnel: [w565 w579] -> w547
              tunnel: [w564 w578] -> w546
              tunnel: w545 -> [w563 w570]
              tunnel: [w563 w568] -> w544
              frame False {
              }
              frame True {
                w576 = T4 {"QueueAction"=enum."TimeOut", "Data"=[], "Data_Raw"=[], "Data_Dark"=[], "Data_Ref"=[], "Device Information"=[], "Numeric Control"=0.0, "Boolean"=FALSE, "Wavelength"=[], "Time"=[], "Time Stamp"=timestamp(0 s since 1904-01-01), "Numeric Control 2"=0.0, "TabControl"=enum."Measure"}  # DataQueue
                w591 = T7 {"QueueAction"=enum."TimeOut", "Numeric 1"=0.0, "Numeric 2"=0.0, "Boolean 1"=FALSE, "Boolean 2"=FALSE, "Spin Program"=[], "Spin Prg v07"=[], "Time Stamp"=timestamp(0 s since 1904-01-01), "TabControl"=enum."Measure"}  # Device Queue
                n217 = call-dynamic "Get_WavelengthAxis.vi"("error in (no error)"=w573, "Avantes in"=w575) -> ("error out"=w572:errorcluster, "lambda"=w567:dbl[unit][], "Avantes out"=w574:refnum<class "Avantes.lvclass">)  [unwired: 7 in]
                n218 = property on="Calculate Frames" class="Bool. (strikt)"() -> ("Value"=w583:bool)  [unwired: 2 in, 2 out]
                n219 = property on="Integration Time" class="DigWert (strikt)"() -> ("Value"=w588:dbl[unit])  [unwired: 2 in, 2 out]
                n220 = Unbundle(w572) -> ("status"=w571:bool)  [unwired: 2 out]
                n221 = node(w588) -> (w587:dbl)
                n222 = Bundle By Name(cluster=w591, "QueueAction"=DeviceQueue_Action."Spectrometer_SetIntegrationTime", "Numeric 1"=w587, "Boolean 1"=w583) -> (w585:T7)
                n223 = property on="Frames" class="DigWert (strikt)"() -> ("Value"=w582:i32)  [unwired: 2 in, 2 out]
                n224 = property on="Error_Spectromter" class="Bool. (strikt)"("Value"=w571) -> ()  [unwired: 2 in, 2 out]
                n225 = Enqueue Element(queue=w590, element=w585, error in (no error)=w573) -> (queue out=w586:refnum<queue>, error out=w580:errorcluster)  [unwired: 1 in, 1 out]
                n226 = Bundle By Name(cluster=w585, "QueueAction"=DeviceQueue_Action."Spectrometer_SetFrames", "Numeric 1"=w582) -> (w581:T7)
                n227 = Bundle By Name(cluster=w576, "QueueAction"=DataQueue_Action."Set_Wavelength", "Wavelength"=w567) -> (w577:T4)
                n228 = Enqueue Element(queue=w570, element=w577) -> (queue out=w568:refnum<queue>)  [unwired: 2 in, 2 out]
                n229 = Enqueue Element(queue=w586, element=w581, error in (no error)=w580) -> (queue out=w579:refnum<queue>, error out=w578:errorcluster)  [unwired: 1 in, 1 out]
              }
            }
            n230 = Bundle By Name(cluster=w556, "Abstract_CCD.lvclass"=w551) -> (w550:T3)
          }
          frame "Spectrometer_Close" {
            n231 = Unbundle By Name(w596) -> ("Abstract_CCD.lvclass"=w599:refnum<class "Abstract_CCD.lvclass">)
            n232 = flat-sequence {
              tunnel: [refnum<class "Abstract_CCD.lvclass"> refnum ("Abstract_CCD.lvclass")] -> w593
              tunnel: w592 -> [_]
              frame #0 {
              }
            }
            n233 = call-dynamic "Close.vi"("error in (no error)"=w598, "Abstract_CCD in"=w599) -> ("error out"=w592:errorcluster)  [unwired: 8 in, 1 out]
            n234 = Bundle By Name(cluster=w596, "Abstract_CCD.lvclass"=w593) -> (w595:T3)
          }
          frame "Spectrometer_Measure" {
            w613 = T4 {"QueueAction"=enum."TimeOut", "Data"=[], "Data_Raw"=[], "Data_Dark"=[], "Data_Ref"=[], "Device Information"=[], "Numeric Control"=0.0, "Boolean"=FALSE, "Wavelength"=[], "Time"=[], "Time Stamp"=timestamp(0 s since 1904-01-01), "Numeric Control 2"=0.0, "TabControl"=enum."Measure"}  # DataQueue
            n235 = Unbundle By Name(w608) -> ("Abstract_CCD.lvclass"=w612:refnum<class "Abstract_CCD.lvclass">)
            n236 = call-dynamic "Measure.vi"("error in (no error)"=w610, "Abstract_CCD in"=w612) -> ("error out"=w609:errorcluster, "Data Raw"=w603:T11, "Data"=w604:T11, "Darkspec"=w602:T11, "Time"=w601:dbl[])  [unwired: 3 in, 2 out]
            n237 = Bundle By Name(cluster=w613, "QueueAction"=DataQueue_Action."TimeOut", "Data"=w604, "Data_Raw"=w603, "Data_Dark"=w602, "Time"=w601) -> (w614:T4)
            n238 = Enqueue Element(queue=w607, element=w614) -> (queue out=w606:refnum<queue>)  [unwired: 2 in, 2 out]
          }
          frame "Spectrometer_Preview" {
            w629 = T4 {"QueueAction"=enum."TimeOut", "Data"=[], "Data_Raw"=[], "Data_Dark"=[], "Data_Ref"=[], "Device Information"=[], "Numeric Control"=0.0, "Boolean"=FALSE, "Wavelength"=[], "Time"=[], "Time Stamp"=timestamp(0 s since 1904-01-01), "Numeric Control 2"=0.0, "TabControl"=enum."Measure"}  # DataQueue
            n239 = Unbundle By Name(w617) -> ("Abstract_CCD.lvclass"=w634:refnum<class "Abstract_CCD.lvclass">)
            n240 = call-dynamic "Get_Frames.vi"("error in (no error)"=w633, "Abstract_CCD in"=w634) -> ("error out"=w635:errorcluster, "Numeric"=w621:i32, "Abstract_CCD out"=w636:refnum<class "Abstract_CCD.lvclass">)  [unwired: 7 in]
            n241 = call-dynamic "Set_Frames.vi"("error in (no error)"=w635, "Frames"=1, "Abstract_CCD in"=w636) -> ("error out"=w632:errorcluster, "Abstract_CCD out"=w637:refnum<class "Abstract_CCD.lvclass">)  [unwired: 7 in]
            n242 = call-dynamic "Measure.vi"("error in (no error)"=w632, "Abstract_CCD in"=w637) -> ("error out"=w623:errorcluster, "Data Raw"=w626:T11, "Abstract_CCD out"=w622:refnum<class "Abstract_CCD.lvclass">)  [unwired: 3 in, 4 out]
            n243 = property on="Preview" class="Bool. (strikt)"() -> ("Value"=w624:bool)  [unwired: 2 in, 2 out]
            n244 = call-dynamic "Set_Frames.vi"("error in (no error)"=w623, "Frames"=w621, "Abstract_CCD in"=w622) -> ("error out"=w620:errorcluster, "Abstract_CCD out"=w615:refnum<class "Abstract_CCD.lvclass">)  [unwired: 7 in]
            n245 = case shown="True" w624 {
              tunnel: [w638 w640] -> w619
              tunnel: w618 -> [w638 w639]
              frame False {
              }
              frame True {
                w642 = T7 {"QueueAction"=enum."TimeOut", "Numeric 1"=0.0, "Numeric 2"=0.0, "Boolean 1"=FALSE, "Boolean 2"=FALSE, "Spin Program"=[], "Spin Prg v07"=[], "Time Stamp"=timestamp(0 s since 1904-01-01), "TabControl"=enum."Measure"}  # Device Queue
                n246 = Bundle By Name(cluster=w642, "QueueAction"=DeviceQueue_Action."Spectrometer_Preview") -> (w641:T7)
                n247 = Enqueue Element(queue=w639, element=w641) -> (queue out=w640:refnum<queue>)  [unwired: 2 in, 2 out]
              }
            }
            n248 = Bundle By Name(cluster=w629, "Data_Raw"=w626, "QueueAction"=DataQueue_Action."Spectrometer_Measure") -> (w630:T4)
            n249 = Enqueue Element(queue=w628, element=w630) -> (queue out=w627:refnum<queue>)  [unwired: 2 in, 2 out]
            n250 = Bundle By Name(cluster=w617, "Abstract_CCD.lvclass"=w615) -> (w616:T3)
          }
          frame "Spectrometer_SetIntegrationTime" {
            n251 = Unbundle By Name(w652) -> ("Numeric 1"=w654:dbl)
            n252 = Unbundle By Name(w646) -> ("Abstract_CCD.lvclass"=w656:refnum<class "Abstract_CCD.lvclass">)
            n253 = Unbundle By Name(w652) -> ("Boolean 1"=w651:bool)
            n254 = node(w654) -> (w653:dbl[unit])
            n255 = call-dynamic "Set_ExposureTime.vi"("error in (no error)"=w655, "Exposure Time"=w653, "Abstract_CCD in"=w656) -> ("error out"=w659:errorcluster, "Abstract_CCD out"=w658:refnum<class "Abstract_CCD.lvclass">)  [unwired: 7 in]
            n256 = call-dynamic "Get_FrameRate.vi"("error in (no error)"=w659, "Abstract_CCD in"=w658) -> ("error out"=w647:errorcluster, "Frame Rate"=w650:dbl[unit], "Abstract_CCD out"=w645:refnum<class "Abstract_CCD.lvclass">)  [unwired: 7 in]
            "Frame Rate" <- w650
            n257 = Bundle By Name(cluster=w646, "Abstract_CCD.lvclass"=w645) -> (w644:T3)
            n258 = case shown="True" w651 {
              tunnel: w650 -> [_ w668]
              tunnel: w649 -> [w660 w662]
              tunnel: [w660 w661] -> w648
              frame False {
              }
              frame True {
                w666 = T7 {"QueueAction"=enum."TimeOut", "Numeric 1"=0.0, "Numeric 2"=0.0, "Boolean 1"=FALSE, "Boolean 2"=FALSE, "Spin Program"=[], "Spin Prg v07"=[], "Time Stamp"=timestamp(0 s since 1904-01-01), "TabControl"=enum."Measure"}  # Device Queue
                n259 = property on="Program Spin Coater\nSpeed (rpm)          Time (s)" class="Arr (strikt)"() -> ("Value"=w671:dbl[][])  [unwired: 2 in, 2 out]
                n260 = property on="Seconds to Spin Start" class="DigWert (strikt)"() -> ("Value"=w670:dbl[unit])  [unwired: 2 in, 2 out]
                n261 = property on="Seconds after Spin Stop" class="DigWert (strikt)"() -> ("Value"=w669:dbl[unit])  [unwired: 2 in, 2 out]
                n262 = call "CalculateFrames.vi"("Program Spin Coater\nSpeed (rpm)          Time (s)"=w671, "Seconds End"=w669, "Seconds Start"=w670, "Frame Rate"=w668) -> ("Time"=w667:dbl, "Frames"=w663:i32)  [unwired: 6 in]
                n263 = property on="Overall Time" class="DigWert (strikt)"("Value"=w667) -> ()  [unwired: 2 in, 2 out]
                n264 = Bundle By Name(cluster=w666, "QueueAction"=DeviceQueue_Action."Spectrometer_SetFrames", "Numeric 1"=w663) -> (w665:T7)
                n265 = Enqueue Element(queue=w662, element=w665) -> (queue out=w661:refnum<queue>)  [unwired: 2 in, 2 out]
              }
            }
          }
          frame "Spectrometer_SetFrames" {
            n266 = Unbundle By Name(w673) -> ("Abstract_CCD.lvclass"=w678:refnum<class "Abstract_CCD.lvclass">)
            n267 = Unbundle By Name(w681) -> ("Numeric 1"=w675:dbl)
            n268 = property on="Frames" class="DigWert (strikt)"("Value"=w675) -> ()  [unwired: 2 in, 2 out]
            n269 = call-dynamic "Set_Frames.vi"("error in (no error)"=w677, "Frames"=w675, "Abstract_CCD in"=w678) -> ("error out"=w676:errorcluster, "Abstract_CCD out"=w672:refnum<class "Abstract_CCD.lvclass">)  [unwired: 7 in]
            n270 = Bundle By Name(cluster=w673, "Abstract_CCD.lvclass"=w672) -> (w674:T3)
          }
          frame "Spectrometer_SetDarkspec" {
            w689 = T4 {"QueueAction"=enum."TimeOut", "Data"=[], "Data_Raw"=[], "Data_Dark"=[], "Data_Ref"=[], "Device Information"=[], "Numeric Control"=0.0, "Boolean"=FALSE, "Wavelength"=[], "Time"=[], "Time Stamp"=timestamp(0 s since 1904-01-01), "Numeric Control 2"=0.0, "TabControl"=enum."Measure"}  # DataQueue
            n271 = Unbundle By Name(w684) -> ("Abstract_CCD.lvclass"=w701:refnum<class "Abstract_CCD.lvclass">)
            n272 = property on="Frames for Dark/Ref" class="DigWert (strikt)"() -> ("Value"=w691:dbl)  [unwired: 2 in, 2 out]
            n273 = call-dynamic "Get_Frames.vi"("error in (no error)"=w693, "Abstract_CCD in"=w701) -> ("error out"=w698:errorcluster, "Numeric"=w699:i32, "Abstract_CCD out"=w700:refnum<class "Abstract_CCD.lvclass">)  [unwired: 7 in]
            n274 = call-dynamic "Set_Frames.vi"("error in (no error)"=w698, "Frames"=w691, "Abstract_CCD in"=w700) -> ("error out"=w697:errorcluster, "Abstract_CCD out"=w694:refnum<class "Abstract_CCD.lvclass">)  [unwired: 7 in]
            n275 = call-dynamic "Measure.vi"("error in (no error)"=w697, "Abstract_CCD in"=w694) -> ("error out"=w696:errorcluster, "Data Raw"=w686:T11, "Abstract_CCD out"=w695:refnum<class "Abstract_CCD.lvclass">)  [unwired: 3 in, 4 out]
            n276 = call-dynamic "Set_Frames.vi"("error in (no error)"=w696, "Frames"=w699, "Abstract_CCD in"=w695) -> ("error out"=w692:errorcluster, "Abstract_CCD out"=w682:refnum<class "Abstract_CCD.lvclass">)  [unwired: 7 in]
            n277 = Bundle By Name(cluster=w689, "QueueAction"=DataQueue_Action."Set_Dark", "Data_Dark"=w686) -> (w690:T4)
            n278 = Enqueue Element(queue=w688, element=w690) -> (queue out=w685:refnum<queue>)  [unwired: 2 in, 2 out]
            n279 = Bundle By Name(cluster=w684, "Abstract_CCD.lvclass"=w682) -> (w683:T3)
          }
          frame "Spectrometer_SetReference" {
            w710 = T4 {"QueueAction"=enum."TimeOut", "Data"=[], "Data_Raw"=[], "Data_Dark"=[], "Data_Ref"=[], "Device Information"=[], "Numeric Control"=0.0, "Boolean"=FALSE, "Wavelength"=[], "Time"=[], "Time Stamp"=timestamp(0 s since 1904-01-01), "Numeric Control 2"=0.0, "TabControl"=enum."Measure"}  # DataQueue
            n280 = Unbundle By Name(w705) -> ("Abstract_CCD.lvclass"=w722:refnum<class "Abstract_CCD.lvclass">)
            n281 = property on="Frames for Dark/Ref" class="DigWert (strikt)"() -> ("Value"=w712:dbl)  [unwired: 2 in, 2 out]
            n282 = call-dynamic "Get_Frames.vi"("error in (no error)"=w714, "Abstract_CCD in"=w722) -> ("error out"=w719:errorcluster, "Numeric"=w720:i32, "Abstract_CCD out"=w721:refnum<class "Abstract_CCD.lvclass">)  [unwired: 7 in]
            n283 = call-dynamic "Set_Frames.vi"("error in (no error)"=w719, "Frames"=w712, "Abstract_CCD in"=w721) -> ("error out"=w718:errorcluster, "Abstract_CCD out"=w715:refnum<class "Abstract_CCD.lvclass">)  [unwired: 7 in]
            n284 = call-dynamic "Measure.vi"("error in (no error)"=w718, "Abstract_CCD in"=w715) -> ("error out"=w717:errorcluster, "Data Raw"=w707:T11, "Abstract_CCD out"=w716:refnum<class "Abstract_CCD.lvclass">)  [unwired: 3 in, 4 out]
            n285 = call-dynamic "Set_Frames.vi"("error in (no error)"=w717, "Frames"=w720, "Abstract_CCD in"=w716) -> ("error out"=w713:errorcluster, "Abstract_CCD out"=w703:refnum<class "Abstract_CCD.lvclass">)  [unwired: 7 in]
            n286 = Bundle By Name(cluster=w710, "QueueAction"=DataQueue_Action."Set_Ref", "Data_Ref"=w707) -> (w711:T4)
            n287 = Enqueue Element(queue=w709, element=w711) -> (queue out=w706:refnum<queue>)  [unwired: 2 in, 2 out]
            n288 = Bundle By Name(cluster=w705, "Abstract_CCD.lvclass"=w703) -> (w704:T3)
          }
          frame "Arduino_Init" {
            w737 = T7 {"QueueAction"=enum."TimeOut", "Numeric 1"=0.0, "Numeric 2"=0.0, "Boolean 1"=FALSE, "Boolean 2"=FALSE, "Spin Program"=[], "Spin Prg v07"=[], "Time Stamp"=timestamp(0 s since 1904-01-01), "TabControl"=enum."Measure"}  # Device Queue
            n289 = call-poly "VISA Configure Serial Port"("VISA resource name"="Port Arduino", "baud rate (9600)"=u32 115200, "error in (no error)"=w743) -> ("VISA resource name out"=w739:refnum<visa-resource-name>, "error out"=w726:errorcluster)  [unwired: 11 in]
            n290 = Unbundle(w726) -> ("status"=w725:bool)  [unwired: 2 out]
            n291 = Not(x=w725) -> (.not. x?=w724:bool)
            n292 = property on="Arduino" class="Bool. (strikt)"("Value"=w724) -> ()  [unwired: 2 in, 2 out]
            n293 = property on="Program Spin Coater\nSpeed (rpm)          Time (s)" class="Arr (strikt)"() -> ("Value"=w732:dbl[][])  [unwired: 2 in, 2 out]
            n294 = Bundle By Name(cluster=w737, "QueueAction"=DeviceQueue_Action."Arduino_LoadProgram", "Spin Program"=dbl[][] []) -> (w733:T7)
            n295 = Enqueue Element(queue=w735, element=w733, error in (no error)=w726) -> (queue out=w731:refnum<queue>, error out=w730:errorcluster)  [unwired: 1 in, 1 out]
            n296 = Bundle By Name(cluster=w733, "Spin Program"=w732) -> (w729:T7)
            n297 = Bundle By Name(cluster=w740, "Port Arduino"=w739) -> (w738:T3)
            n298 = Enqueue Element(queue=w731, element=w729, error in (no error)=w730) -> (queue out=w728:refnum<queue>, error out=w727:errorcluster)  [unwired: 1 in, 1 out]
          }
          frame "Arduino_Close" {
            n299 = Unbundle By Name(w747) -> ("Port Arduino"=w751:refnum<visa-resource-name>)
            n300 = property on="Arduino" class="Bool. (strikt)"("Value"=FALSE ("Arduino")) -> ()  [unwired: 2 in, 2 out]
            n301 = VISA Close(VISA resource name=w751, error in (no error)=w750) -> (error out=w749:errorcluster)
          }
          frame "Arduino_LoadProgram" {
            n302 = Unbundle By Name(w754) -> ("Spin Program"=w753:dbl[][])
            n303 = Unbundle By Name(w756) -> ("Port Arduino"=w758:refnum<visa-resource-name>)
            n304 = call "SpinCoaterArray2String.vi"("Program Spin Coater\nSpeed (rpm)          Time (s)"=w753) -> ("remote control String"=w752:string)  [unwired: 4 in]
            n305 = VISA Write(VISA resource name=w758, write buffer=w752, error in (no error)=w759) -> (error out=w755:errorcluster)  [unwired: 2 out]
          }
          frame "Arduino_StartProgram" {
            n306 = Unbundle By Name(w766) -> ("Port Arduino"=w765:refnum<visa-resource-name>)
            n307 = VISA Write(VISA resource name=w765, write buffer="run", error in (no error)=w763) -> (error out=w762:errorcluster)  [unwired: 2 out]
          }
          frame "Arduino_SetSpeed" {
            n308 = Unbundle By Name(w776) -> ("Numeric 1"=w774:dbl)
            n309 = Unbundle By Name(w778) -> ("Port Arduino"=w777:refnum<visa-resource-name>)
            n310 = To Unsigned Long Integer(number=w774) -> (unsigned 32bit integer=w773:u32)
            n311 = Number To Decimal String(number=w773) -> (decimal integer string=w772:string)  [unwired: 1 in]
            n312 = Concatenate Strings("!spe" ("string"), w772) -> (w770:string)
            n313 = VISA Write(VISA resource name=w777, write buffer=w770, error in (no error)=w775) -> (error out=w769:errorcluster)  [unwired: 2 out]
          }
          frame "Arduino_SetMillis" {
            n314 = Unbundle By Name(w782) -> ("Numeric 1"=w790:dbl)
            n315 = Unbundle By Name(w780) -> ("Port Arduino"=w791:refnum<visa-resource-name>)
            n316 = To Unsigned Long Integer(number=w790) -> (unsigned 32bit integer=w789:u32)
            n317 = Number To Decimal String(number=w789) -> (decimal integer string=w788:string)  [unwired: 1 in]
            n318 = Concatenate Strings("!mil" ("string"), w788) -> (w786:string)
            n319 = VISA Write(VISA resource name=w791, write buffer=w786, error in (no error)=w785) -> (error out=w783:errorcluster)  [unwired: 2 out]
          }
          frame "Arduino_StopSpin" {
            n320 = Unbundle By Name(w795) -> ("Port Arduino"=w794:refnum<visa-resource-name>)
            n321 = VISA Write(VISA resource name=w794, write buffer="abo", error in (no error)=w796) -> (error out=w792:errorcluster)  [unwired: 2 out]
          }
          frame "Measure_InSitu" {
            w809 = T4 {"QueueAction"=enum."TimeOut", "Data"=[], "Data_Raw"=[], "Data_Dark"=[], "Data_Ref"=[], "Device Information"=[], "Numeric Control"=0.0, "Boolean"=FALSE, "Wavelength"=[], "Time"=[], "Time Stamp"=timestamp(0 s since 1904-01-01), "Numeric Control 2"=0.0, "TabControl"=enum."Measure"}  # DataQueue
            w818 = T4 {"QueueAction"=enum."TimeOut", "Data"=[], "Data_Raw"=[], "Data_Dark"=[], "Data_Ref"=[], "Device Information"=[], "Numeric Control"=0.0, "Boolean"=FALSE, "Wavelength"=[], "Time"=[], "Time Stamp"=timestamp(0 s since 1904-01-01), "Numeric Control 2"=0.0, "TabControl"=enum."Measure"}  # DataQueue
            n322 = flat-sequence {
              tunnel: w827 -> [w839]
              tunnel: [w838] -> w832
              tunnel: [w837] -> w831
              tunnel: [w836] -> w830
              tunnel: w828 -> [w835]
              tunnel: [w835] -> w829
              tunnel: w832 -> [w849]
              tunnel: w831 -> [w840]
              tunnel: w830 -> [w841]
              tunnel: w829 -> [w848]
              tunnel: [w845] -> w826
              tunnel: [w844] -> w825
              tunnel: [w843] -> w824
              tunnel: [w842] -> w823
              tunnel: [w841] -> w821
              tunnel: [w840] -> w820
              tunnel: w826 -> [w858]
              tunnel: w825 -> [w860]
              tunnel: w824 -> [w859]
              tunnel: w823 -> [w862]
              tunnel: w822 -> [w861]
              tunnel: [w857] -> w812
              tunnel: w821 -> [w856]
              tunnel: w820 -> [w855]
              tunnel: [w854] -> w817
              tunnel: [w853] -> w816
              tunnel: [w852] -> w805
              tunnel: [w851] -> w813
              tunnel: [w850] -> w815
              frame #0 {
                n323 = Unbundle By Name(w839) -> ("Abstract_CCD.lvclass"=w838:refnum<class "Abstract_CCD.lvclass">, "Port Arduino"=w837:refnum<visa-resource-name>)
                n324 = property on="Seconds to Spin Start" class="DigWert (strikt)"() -> ("Value"=w834:dbl[unit])  [unwired: 2 in, 2 out]
                n325 = node(w834) -> (w836:dbl)
              }
              frame #1 {
                n326 = Greater Than 0?(x=w841) -> (x > 0?=w842:bool)
                n327 = call-dynamic "Get_Frames.vi"("error in (no error)"=w848, "Abstract_CCD in"=w849) -> ("error out"=w843:errorcluster, "Numeric"=w847:i32, "Abstract_CCD out"=w844:refnum<class "Abstract_CCD.lvclass">)  [unwired: 7 in]
                n328 = call "PrepareFrames.vi"("Frames Limit"=30000, "Frames"=w847) -> ("FrameList"=w845:i32[])  [unwired: 9 in]
              }
              frame #2 {
                n329 = case shown="True" w862 {
                  tunnel: w861 -> [w873 w917]
                  tunnel: w860 -> [w875 w921]
                  tunnel: w859 -> [w869 w915]
                  tunnel: w858 -> [w874 w919]
                  tunnel: [w872 w916] -> w857
                  tunnel: w856 -> [w870 w913]
                  tunnel: w855 -> [w868 w914]
                  tunnel: [w867 w912] -> w854
                  tunnel: [w866 w911] -> w853
                  tunnel: [w865 w910] -> w852
                  tunnel: [w864 w909] -> w851
                  tunnel: [w863 w908] -> w850
                  frame True {
                    # "Spectrometer before Spin Coater"
                    n330 = flat-sequence {
                      tunnel: w873 -> [w887]
                      tunnel: [w886] -> w872
                      tunnel: w874 -> [w888]
                      tunnel: w869 -> [w889]
                      tunnel: w875 -> [w890]
                      tunnel: [w885] -> w867
                      tunnel: [w884] -> w866
                      tunnel: [w883] -> w863
                      frame #0 {
                        n331 = for {
                          shift-right: [w893] -> w885
                          shift-left: w890 -> [w906]
                          tunnel: w888 -> [w902] mode=indexing
                          shift-right: [w894] -> w886
                          shift-left: w887 -> [w895]
                          shift-right: [w892] -> w884
                          shift-left: w889 -> [w905]
                          tunnel: [w891] -> w883 mode=indexing
                          w900 = T4 {"QueueAction"=enum."TimeOut", "Data"=[], "Data_Raw"=[], "Data_Dark"=[], "Data_Ref"=[], "Device Information"=[], "Numeric Control"=0.0, "Boolean"=FALSE, "Wavelength"=[], "Time"=[], "Time Stamp"=timestamp(0 s since 1904-01-01), "Numeric Control 2"=0.0, "TabControl"=enum."Measure"}  # DataQueue
                          n332 = Bundle("Numeric Control"=w902, u16 0, u16 1409) -> (w901:cluster{"Numeric Control":i32, u16, u16})  [unwired: 1 in]
                          n333 = call-dynamic "Measure.vi"("error in (no error)"=w905, "Variant"=w901, "Option"=1, "Abstract_CCD in"=w906) -> ("error out"=w892:errorcluster, "Data Raw"=w898:T11, "Abstract_CCD out"=w893:refnum<class "Abstract_CCD.lvclass">, "Time"=w897:dbl[], "Starting Time"=w891:dbl)  [unwired: 1 in, 2 out]
                          n334 = Bundle By Name(cluster=w900, "QueueAction"=DataQueue_Action."Spectrometer_Measure", "Data_Raw"=w898, "Time"=w897) -> (w896:T4)
                          n335 = Enqueue Element(queue=w895, element=w896) -> (queue out=w894:refnum<queue>)  [unwired: 2 in, 2 out]
                        }
                      }
                    }
                    n336 = flat-sequence {
                      tunnel: w870 -> [w877]
                      tunnel: w869 -> [w876]
                      tunnel: [w876] -> w871
                      tunnel: w868 -> [w882]
                      tunnel: w871 -> [w880]
                      tunnel: [w879] -> w864
                      tunnel: [w878] -> w865
                      frame #0 {
                        n337 = Wait (ms)(milliseconds to wait=w877) -> ()  [unwired: 1 out]
                      }
                      frame #1 {
                        n338 = call <vilib>:"High Resolution Relative Seconds.vi"() -> ("relative seconds"=w879:dbl)
                        n339 = VISA Write(VISA resource name=w882, write buffer="run", error in (no error)=w880) -> (error out=w878:errorcluster)  [unwired: 2 out]
                      }
                    }
                  }
                  frame False {
                    # "Spin Coater before Spectrometer"
                    n340 = flat-sequence {
                      tunnel: [w931] -> w922
                      tunnel: w921 -> [w931]
                      tunnel: [w930] -> w920
                      tunnel: w915 -> [w930]
                      tunnel: w919 -> [w929]
                      tunnel: [w929] -> w918
                      tunnel: w913 -> [w928]
                      tunnel: w922 -> [w939]
                      tunnel: w920 -> [w938]
                      tunnel: w918 -> [w937]
                      tunnel: w917 -> [w936]
                      tunnel: [w935] -> w916
                      tunnel: [w934] -> w912
                      tunnel: [w933] -> w911
                      tunnel: [w932] -> w908
                      frame #0 {
                        n341 = Wait (ms)(milliseconds to wait=w928) -> ()  [unwired: 1 out]
                      }
                      frame #1 {
                        n342 = for {
                          shift-right: [w942] -> w934
                          shift-left: w939 -> [w955]
                          tunnel: w937 -> [w951] mode=indexing
                          shift-right: [w943] -> w935
                          shift-left: w936 -> [w944]
                          shift-right: [w941] -> w933
                          shift-left: w938 -> [w954]
                          tunnel: [w940] -> w932 mode=indexing
                          w949 = T4 {"QueueAction"=enum."TimeOut", "Data"=[], "Data_Raw"=[], "Data_Dark"=[], "Data_Ref"=[], "Device Information"=[], "Numeric Control"=0.0, "Boolean"=FALSE, "Wavelength"=[], "Time"=[], "Time Stamp"=timestamp(0 s since 1904-01-01), "Numeric Control 2"=0.0, "TabControl"=enum."Measure"}  # DataQueue
                          n343 = Bundle("Numeric Control"=w951, u16 0, u16 1409) -> (w950:cluster{"Numeric Control":i32, u16, u16})  [unwired: 1 in]
                          n344 = call-dynamic "Measure.vi"("error in (no error)"=w954, "Variant"=w950, "Option"=1, "Abstract_CCD in"=w955) -> ("error out"=w941:errorcluster, "Data Raw"=w947:T11, "Abstract_CCD out"=w942:refnum<class "Abstract_CCD.lvclass">, "Time"=w946:dbl[], "Starting Time"=w940:dbl)  [unwired: 1 in, 2 out]
                          n345 = Bundle By Name(cluster=w949, "QueueAction"=DataQueue_Action."Spectrometer_Measure", "Data_Raw"=w947, "Time"=w946) -> (w945:T4)
                          n346 = Enqueue Element(queue=w944, element=w945) -> (queue out=w943:refnum<queue>)  [unwired: 2 in, 2 out]
                        }
                      }
                    }
                    n347 = flat-sequence {
                      tunnel: w914 -> [w927]
                      tunnel: [w924] -> w909
                      tunnel: [w923] -> w910
                      tunnel: w915 -> [w925]
                      frame #0 {
                        n348 = call <vilib>:"High Resolution Relative Seconds.vi"() -> ("relative seconds"=w924:dbl)
                        n349 = VISA Write(VISA resource name=w927, write buffer="run", error in (no error)=w925) -> (error out=w923:errorcluster)  [unwired: 2 out]
                      }
                    }
                  }
                }
              }
            }
            n350 = Index Array(array=w815, index=0) -> (element=w803:dbl)
            n351 = call-dynamic "Get_DeviceInformation.vi"("error in (no error)"=w816, "Abstract_CCD in"=w817) -> ("error out"=w799:errorcluster, "Array"=w801:string[])  [unwired: 7 in, 1 out]
            n352 = Subtract(x=w803, y=w813) -> (x-y=w802:dbl)
            n353 = property on="StartMeasurement_Button" class="Bool. (strikt)"(error in=w799, "Value"=FALSE ("StartMeasurement_Button")) -> ()  [unwired: 1 in, 2 out]
            n354 = Bundle By Name(cluster=w809, "QueueAction"=DataQueue_Action."Stop_Measurement") -> (w807:T4)
            n355 = Bundle By Name(cluster=w818, "QueueAction"=DataQueue_Action."Transfer_Settings", "Device Information"=w801, "Numeric Control"=w803, "Numeric Control 2"=w802) -> (w811:T4)
            n356 = Merge Errors(w799, w805) -> (w804:errorcluster)
            n357 = Enqueue Element(queue=w812, element=w811) -> (queue out=w810:refnum<queue>)  [unwired: 2 in, 2 out]
            n358 = Enqueue Element(queue=w810, element=w807) -> (queue out=w806:refnum<queue>)  [unwired: 2 in, 2 out]
          }
        }
      }
      frame Error {
        w961 = T14 4 items=["no dialog", "OK message", "continue or stop message", "OK message + warnings", "continue/stop + warnings"] ("type of dialog (OK msg:1)")
        n359 = call <vilib>:"General Error Handler.vi"("type of dialog (OK msg:1)"=w961, "error in (no error)"=w962) -> ("error out"=w960:errorcluster)  [unwired: 9 in, 4 out]
        n360 = call <vilib>:"Clear Errors.vi"("error in (no error)"=w960) -> ("error out"=w959:errorcluster)  [unwired: 5 in, 1 out]
      }
    }
  }
  n361 = Release Queue(queue=w5) -> ()  [unwired: 2 in, 3 out]
  n362 = Release Queue(queue=w6) -> ()  [unwired: 2 in, 3 out]
  n363 = property on="Action" class="Str"("Value"="Measuring" ("Action")) -> ()  [unwired: 2 in, 2 out]
